vi "TAT_Auto.vi"(8 "error in (no error)":errorcluster) -> (0 "error out":errorcluster)   [LabVIEW 2017]
uses:
  Controls/TRIP_VALUS_STATUS.ctl
  <vilib>/Utility/error.llb/DialogType.ctl
  Controls/AUTO_DATA.ctl
  Controls/QUEUE_STATES.ctl
  <vilib>/Utility/miscctls.llb/LVRowAndColumnUnsignedTypeDef.ctl
  Controls/AUTO_St.ctl
  6e3b2da7-da9a-4fdb-b6c6-0a8c66529e34.vi
  da0a1603-3ba1-4d29-b87e-07a202ff7828.vi
  <vilib>/Instr/_visa.llb/VISA Configure Serial Port (Instr).vi
  Global/PLC_to_Auto.vi
  <userlib>/_OpenG.lib/array/array.llb/Search 1D Array (Boolean)__ogtk.vi
  <vilib>/Utility/config.llb/NI_LVConfig.lvlib
panel:
  out "TRIP CAUSE":T1=enum."TRIP FORCE HIGHER FAIL"
  out "TRIP FORCE":u32
  out "RESET FORCE":u32
  out "SYSTEM READY ST 2":bool
  out "CYCLE RUNNING ST 2":bool
  out "LOAD gms":cluster{"X DISTANCE":dbl[], "Y LOAD":dbl[]}(graph) caption="XY Graph - Dark"
  out "TF PART OK SCAN ST2":bool
  out "TF RUNNING PART ST2":string caption="TF RUNNING PART"
  out "LOAD":string
  out "3. POSITION 3 DONE":bool
  out "2. POSITION 2 DONE":bool
  out "1. POSITION 1 DONE":bool
  out "PART PRESENT":bool
  out "STOCK COUNTER":string
  out "MOP OPERATION OK":bool
  out "MOTOR HOME":bool
  out "PART OK ST 1":bool
  out "SYSTEM READY ST 1":bool
  out "CYCLE RUNNING STATION 1":bool
  out "Table":string[][](table)
  out "Scaned 2 Code":string
  out "Scanner 2 Status":bool
  out "mechanisum ok ack":bool
  out "housing ok ack":bool
  out "error out 2":errorcluster
  in  "COUNTER RESET":bool
  out "Load Cell Scaned":string
  out "Load Cell Status":bool
  out "Scanner 1 Status":bool
  out "Scaned 1 Code":string
  out "PLC STATUS":bool
  out "MECHANISUM DATA ST1":string caption="MECHANISUM DATA"
  out "NG COUNTER":string
  out "OK COUNTER":string
  out "CYCLE TIME (Sec)":string
  out "MAIN LOOP STOPED ?":bool
  out "Alarms":string[](array[string])
  out "HOUSING DATA ST1":string caption="HOUSING DATA"
  in  "Stop":bool
  out "DATE/TIME":string
  out "screen name":string
  out "ALARMS:-":string
  out "USER:-":string
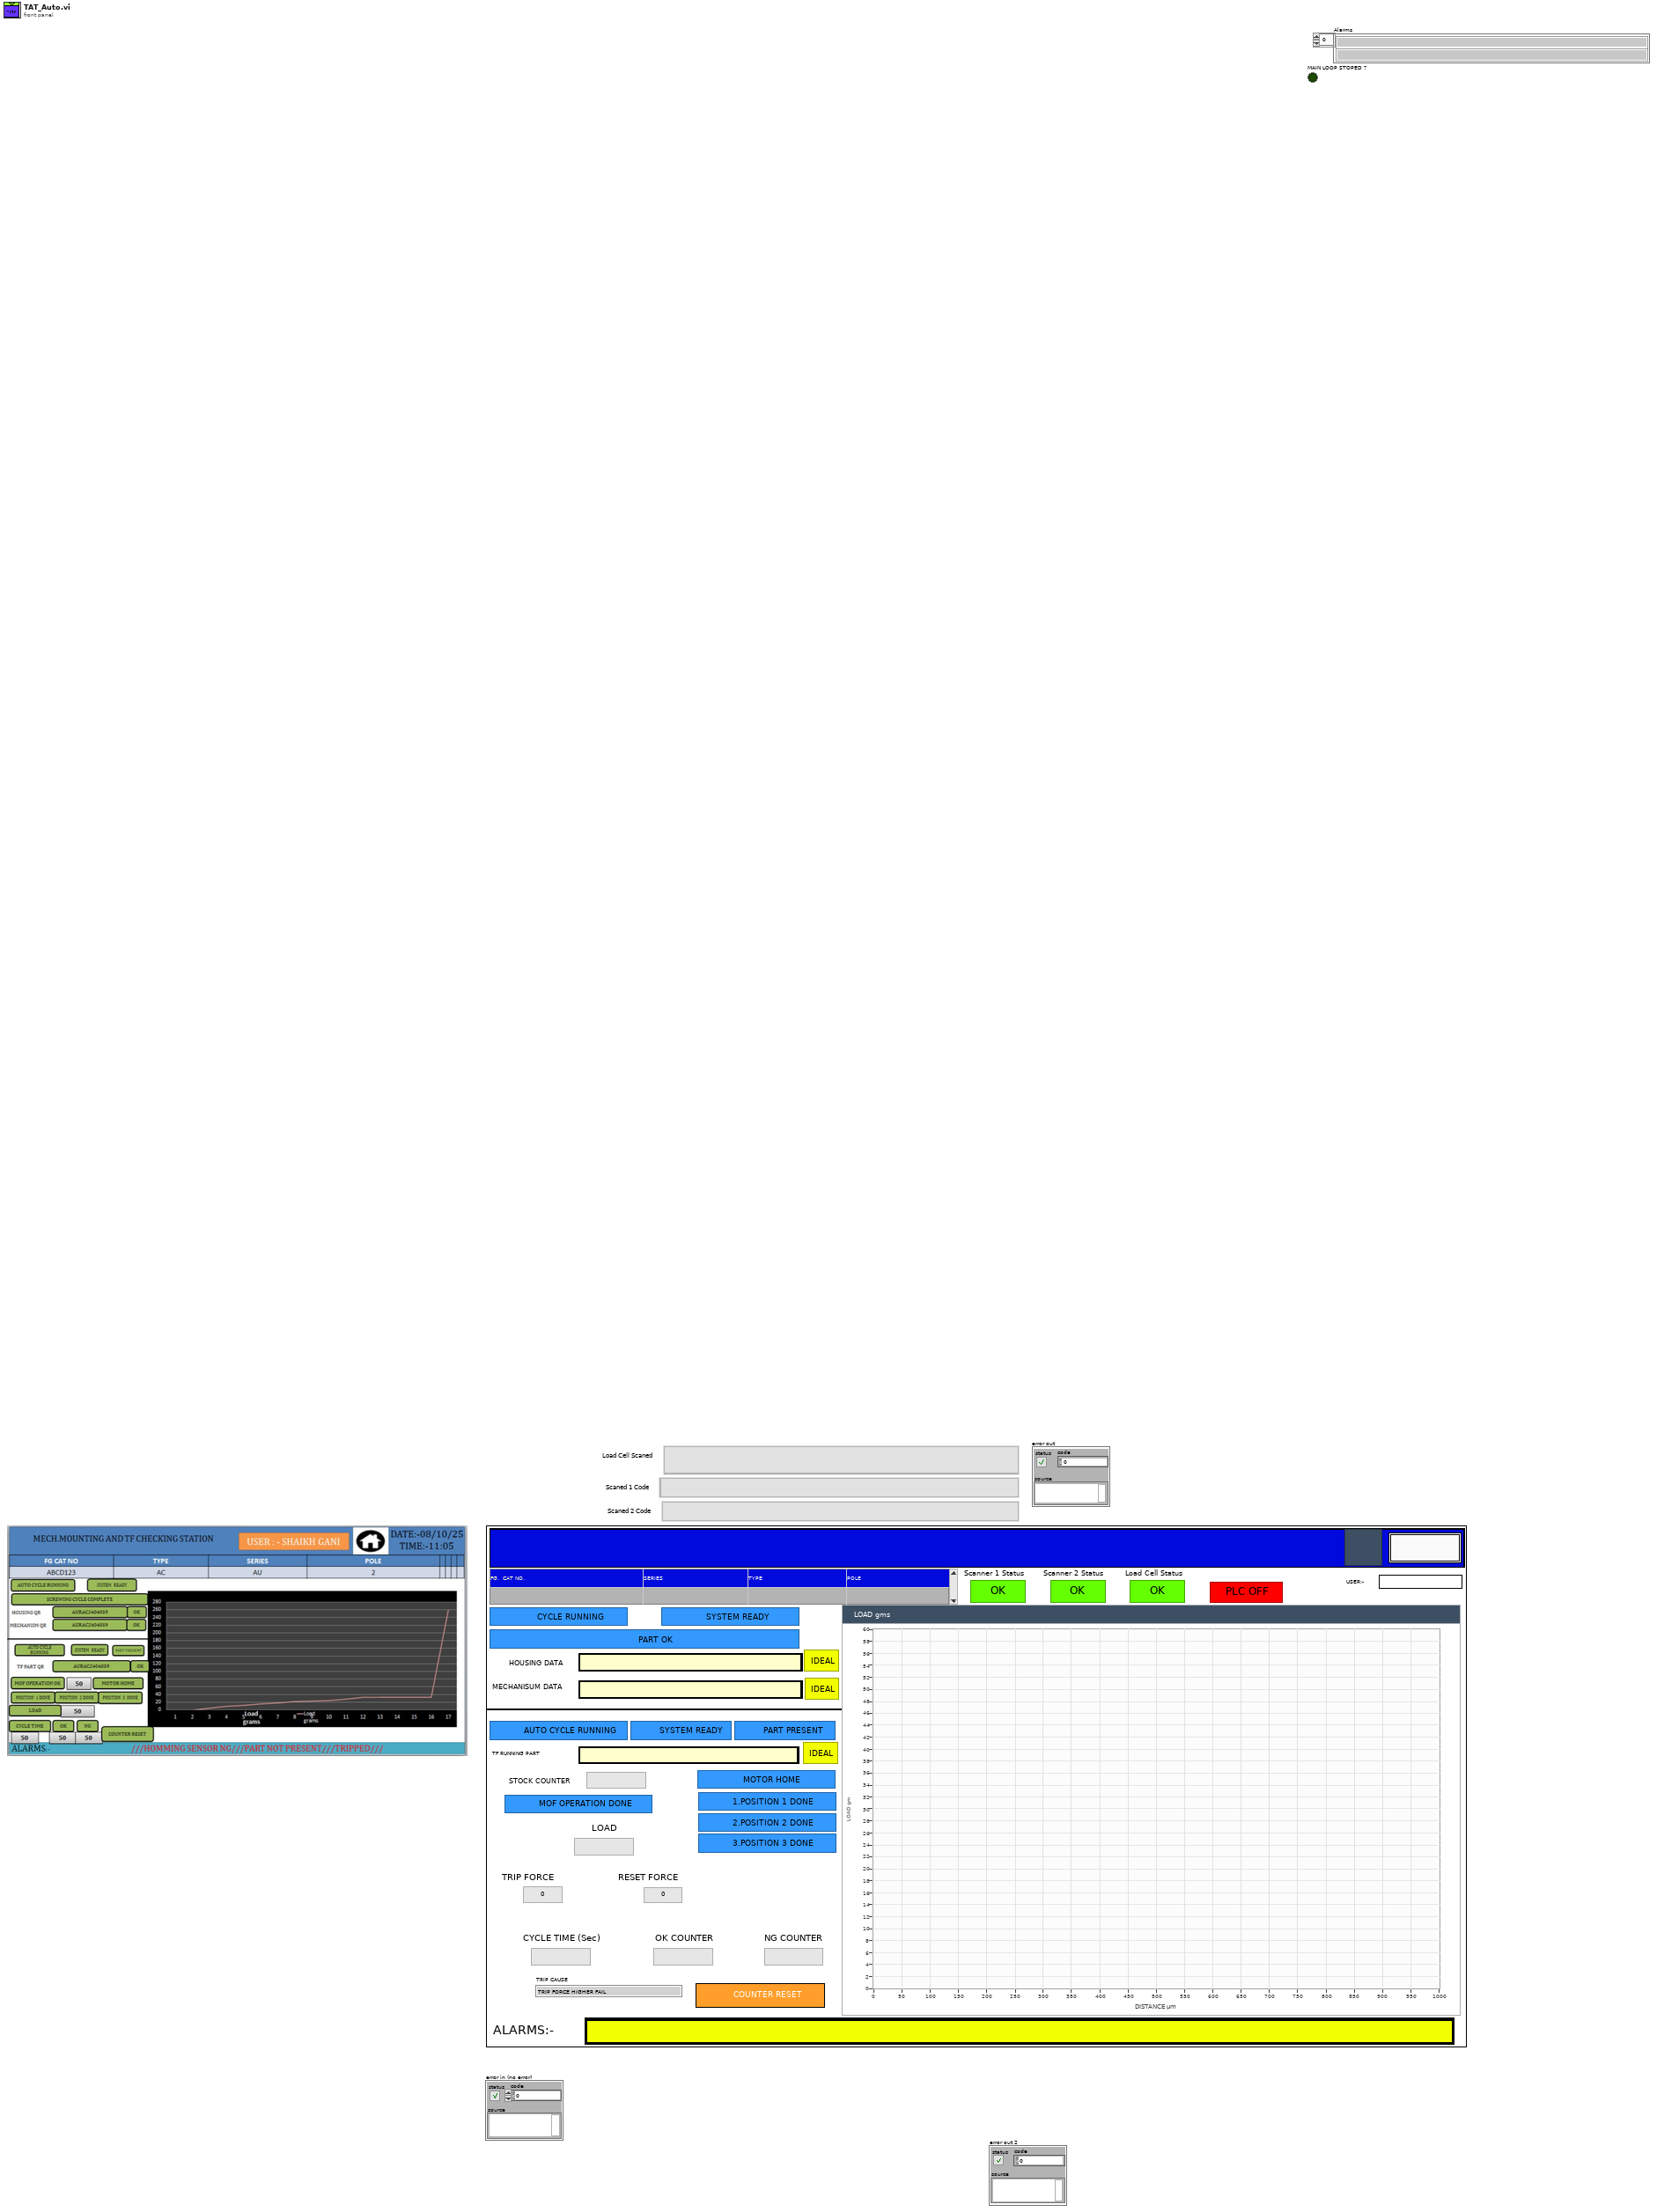
[diagram p1: front panel]
types:
  T1 = typedef "TRIP_VALUS_STATUS.ctl" = enum16{"RESET FORCE HIGHER FAIL", "TRIP FORCE HIGHER FAIL", "TRIP FORCE LOWER FAIL", "IDEAL", "TRIP RESET ACHIVED"}
  T2 = typedef "AUTO_DATA.ctl" = cluster{"SINGLE VARIENT":cluster{"HOUASING":string, "MECHANISUM":string, "VARIENT No.":string, "TYPE":string, "SERIES":string, "POLE":string}, "CYCLE DATA":cluster{"SCANNED HOUSING ST1":string, "SCANNED MECHANISUM ST1":string, "X DISTANCE":dbl[], "Y LOAD":dbl[], "prn DATA":string, "SCANNED HOUSING 1 OK":string[], "SCANNED HOUSING TF ST2":string}, "TF CHECKING PARAMATERS":cluster{"TRIP FORCE MIN":u16, "RESET FORCE MIN":u16, "OFFSET":i16, "TRIP FORCE MAX":u16, "RESET FORCE MAX":u16}, "REFERENCE":cluster{"TRIP FORCE":refnum<vi>, "RESET FORCE":refnum<vi>}}
  T3 = typedef "DialogType.ctl" = u16
  T4 = cluster{"PLC IP ADDRESS":string, "SCAN 1 COM":refnum<visa-resource-name>, "SCAN 2 COM":refnum<visa-resource-name>, "LOAD CELL COM":refnum<visa-resource-name>, "PRINTER IP ADDRESS":string}
  T5 = typedef "QUEUE_STATES.ctl" = enum16{"CREATE Q", "EN Q", "DE Q", "CLOSE Q"}
  T6 = typedef "AUTO_St.ctl" = enum16{"Int", "Int2", "CLUSTER_UPDATE", "WAIT", "AUTO_CYCLE_RUNNING_ST1", "SCAN_STATION_1", "STATION_1_CMPLT_OK", "STATION_1_ABORT_NG", "SCAN_STATION_2", "LOAD CELL PICK UP", "AUTO_CYCLE_COMP_ST2", "AUTO_CYCLE_ABORT_ST2", "PRINT", "CYCLE_DISTANCE FAIL_ST2", "AUTO_CYC_START_ST2", "Error_Handler", "Stop"}
  T7 = typedef "LVRowAndColumnUnsignedTypeDef.ctl" = cluster{"Row":u32, "Column":u32}
  T8 = enum32{"invalid app kind", "Development System", "Run Time System", "Student Edition", "Embedded LabVIEW", "Evaluation", "Custom"}
  T9 = typedef "NI_LVConfig.lvlib/Config Data RefNum.ctl" = refnum<k1>
  T10 = cluster{"HOUASING":string, "MECHANISUM":string, "VARIENT No.":string, "TYPE":string, "SERIES":string, "POLE":string}
  T11 = cluster{"TRIP FORCE MIN":u16, "RESET FORCE MIN":u16, "OFFSET":i16, "TRIP FORCE MAX":u16, "RESET FORCE MAX":u16}
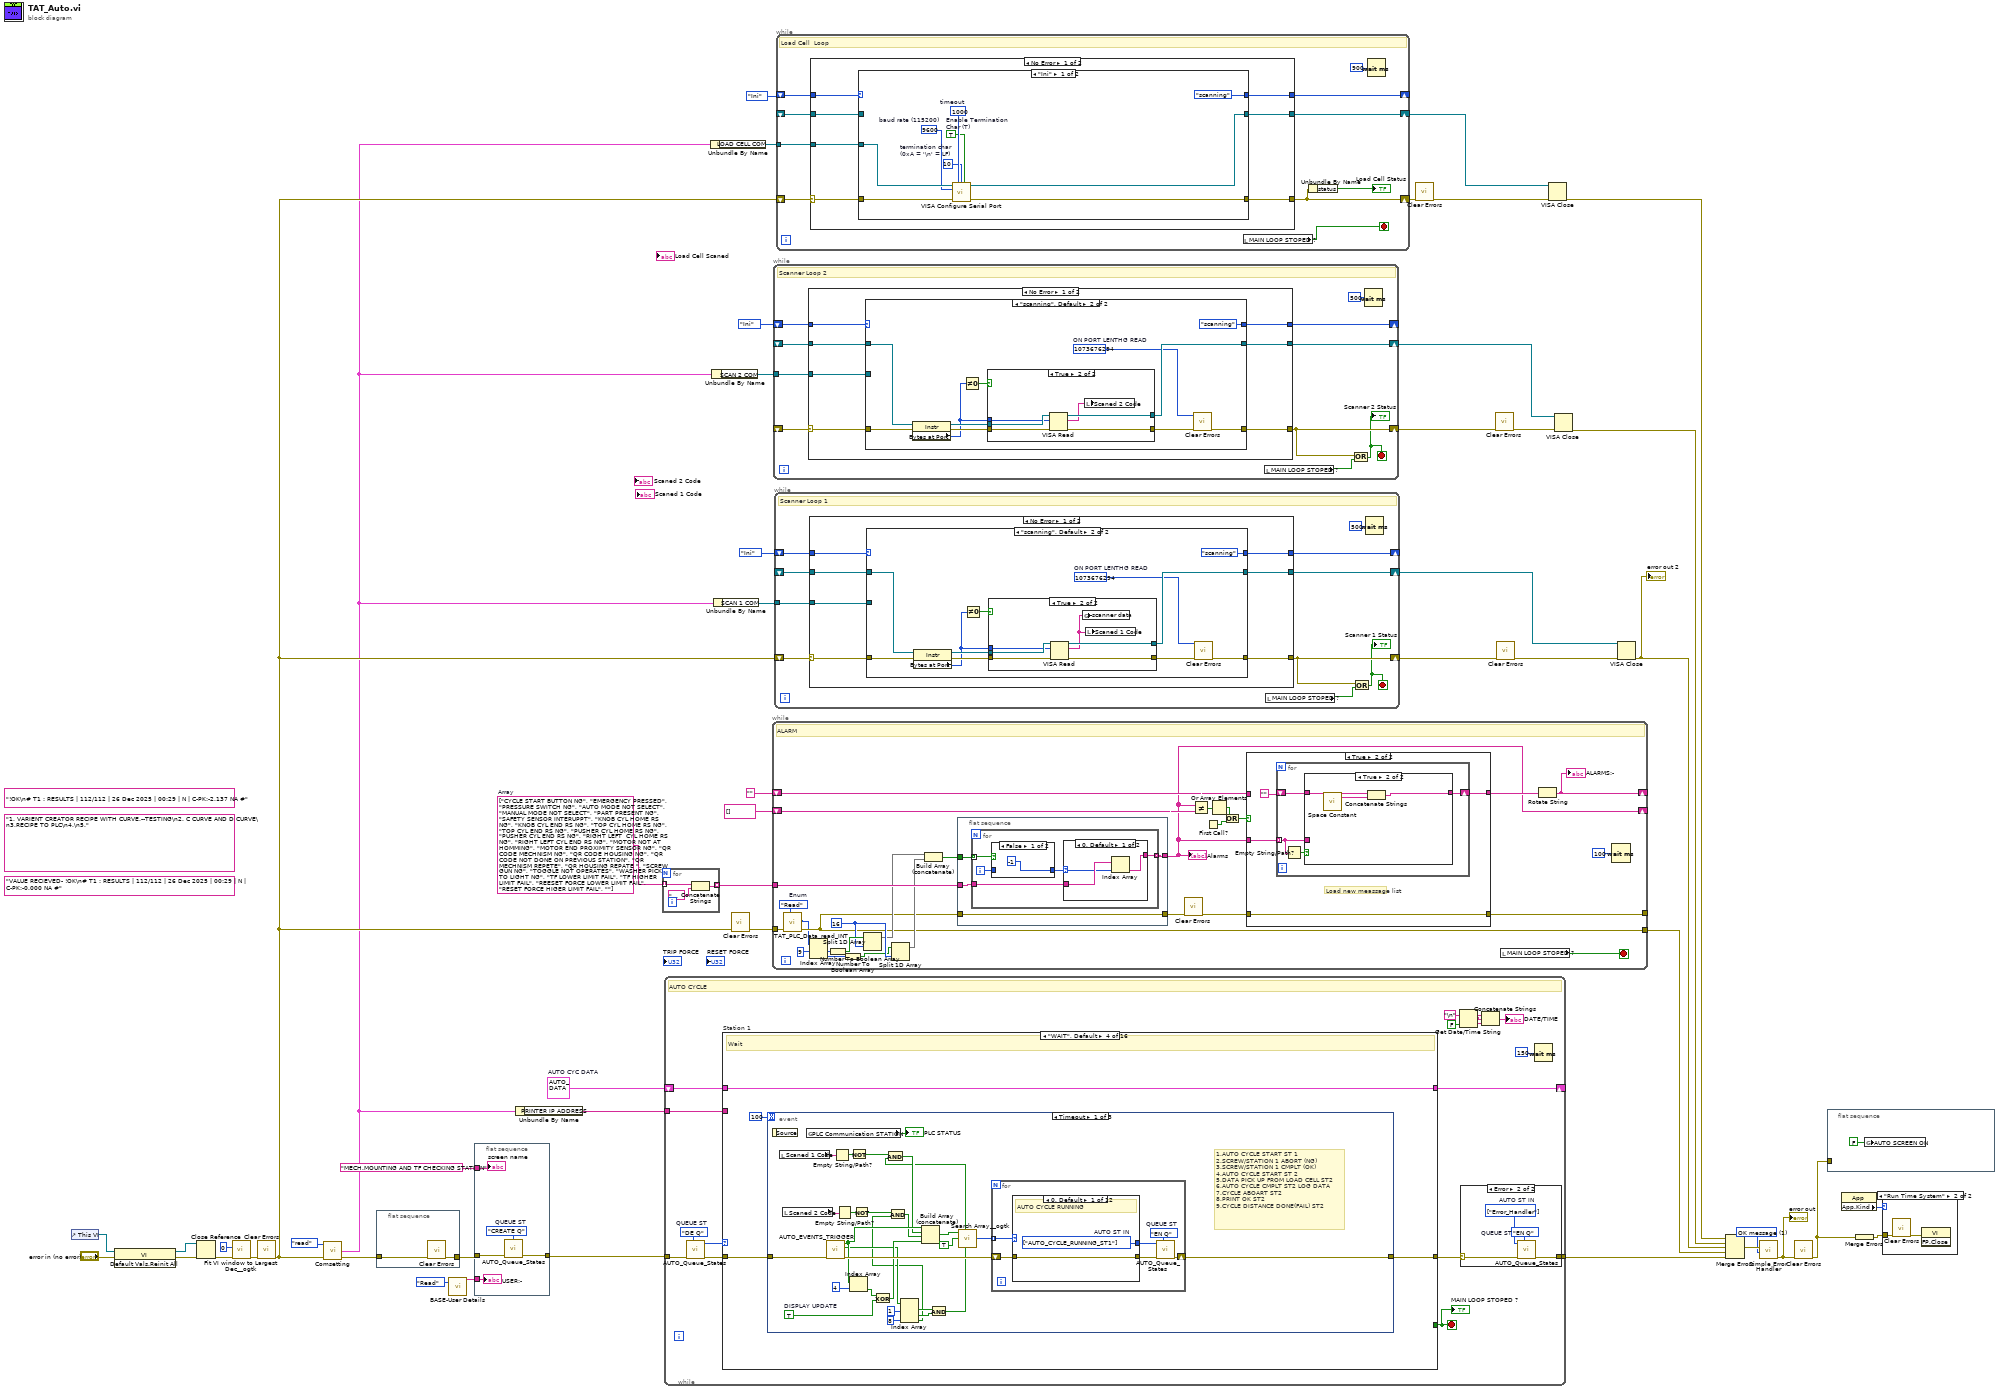
[diagram p0: block diagram]
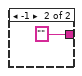
[diagram p2: hidden frame]
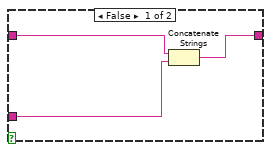
[diagram p5: hidden frame]
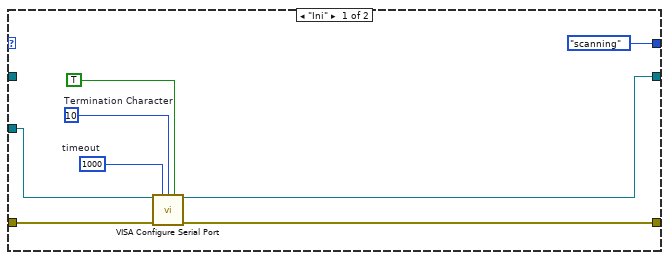
[diagram p7: hidden frame]
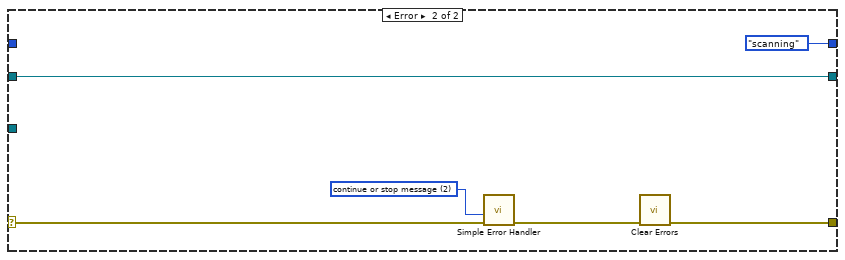
[diagram p9: hidden frame]
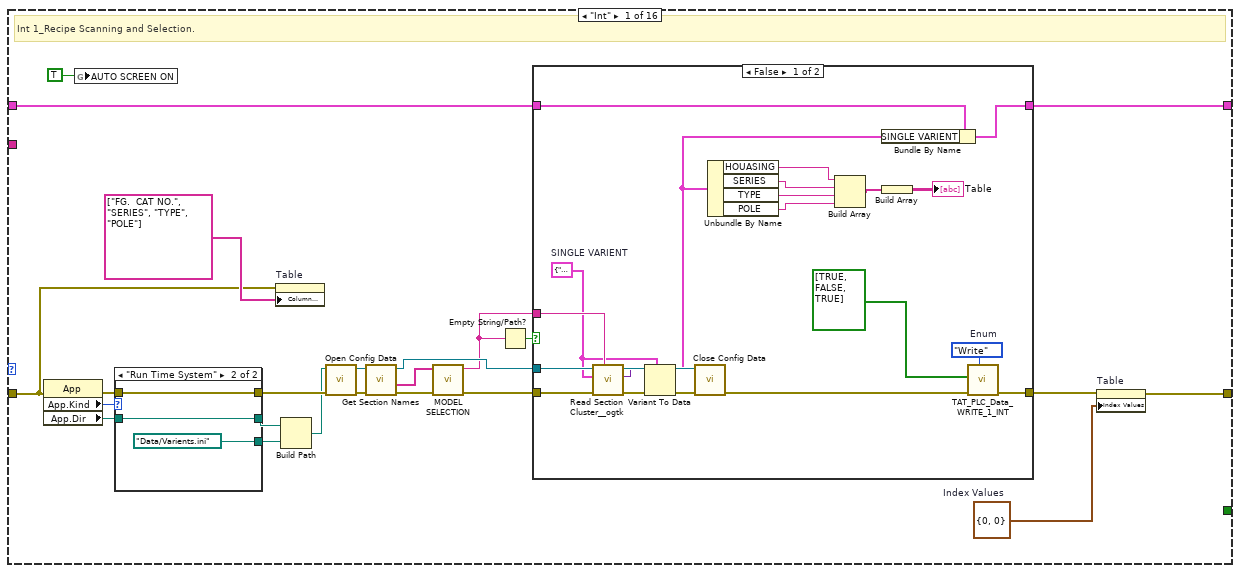
[diagram p11: hidden frame]
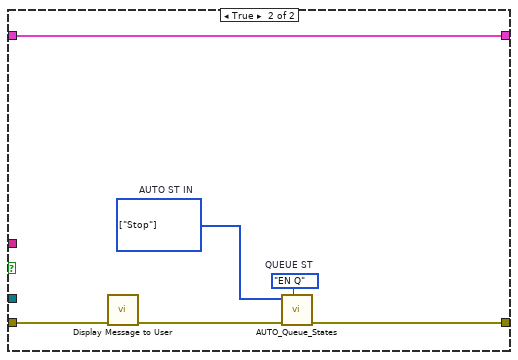
[diagram p12: hidden frame]
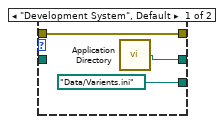
[diagram p13: hidden frame]
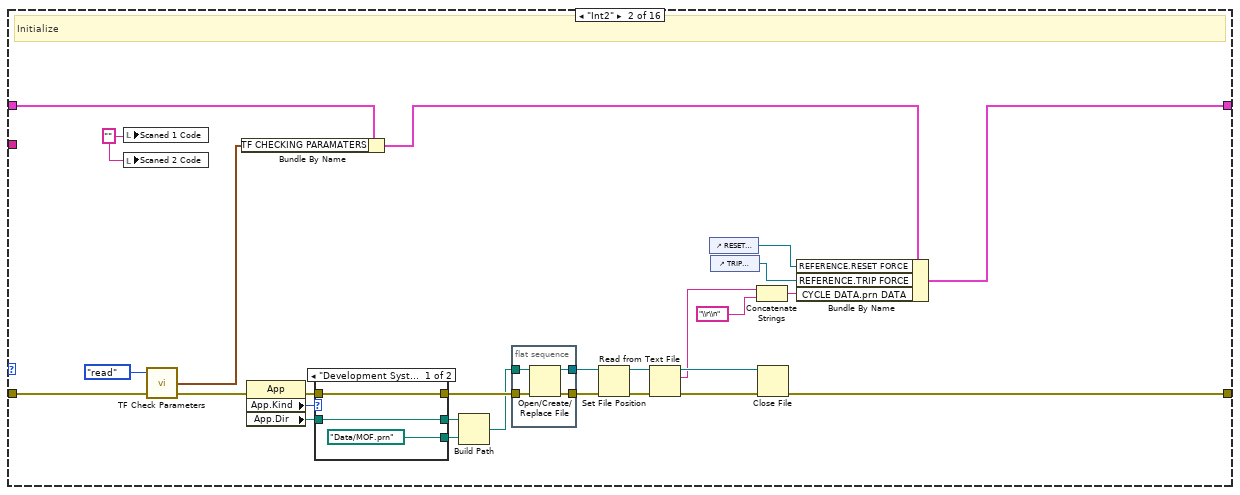
[diagram p14: hidden frame]
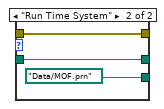
[diagram p15: hidden frame]
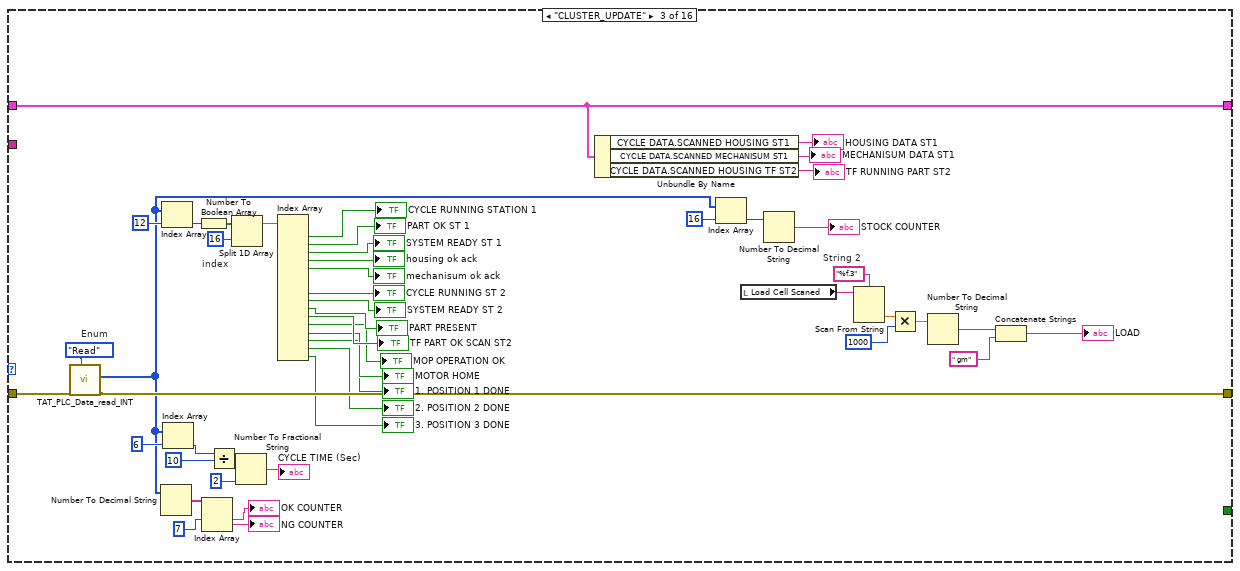
[diagram p16: hidden frame]
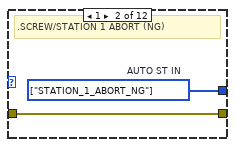
[diagram p17: hidden frame]
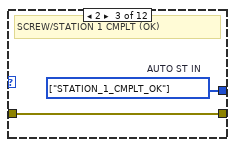
[diagram p18: hidden frame]
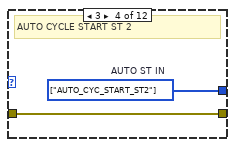
[diagram p19: hidden frame]
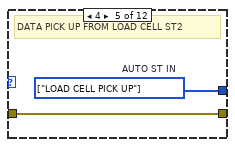
[diagram p20: hidden frame]
diagram:
  w3 = string[] ["CYCLE START BUTTON NG", "EMERGENCY PRESSED", "PRESSURE SWITCH NG", "AUTO MODE NOT SELECT", "MANUAL MODE NOT SELECT", "PART PRESENT NG", "SAFETY SENSOR INTERUPPT", "KNOB CYL HOME RS NG", "KNOB CYL END RS NG", "TOP CYL HOME RS NG", "TOP CYL END RS NG", "PUSHER CYL HOME RS NG", "PUSHER CYL END RS NG", "RIGHT LEFT  CYL HOME RS NG", "RIGHT LEFT CYL END RS NG", "MOTOR NOT AT HOMMING", "MOTOR END PROXIMITY SENSOR NG", "QR CODE MECHNISM NG", "QR CODE HOUSING NG", "QR CODE NOT DONE ON PREVIOUS STATION", "QR MECHNISM REPETE", "QR HOUSING REPATE ", "SCREW GUN NG", "TOGGLE NOT OPERATES", "WASHER PICK TO LIGHT NG", "TF LOWER LIMIT FAIL", "TF HIGHER LIMIT FAIL", "REESET FORCE LOWER LIMIT FAIL", "RESET FORCE HIGER LIMIT FAIL", ""]  # Array
  w23 = T2 {"SINGLE VARIENT"={"HOUASING"="", "MECHANISUM"="", "VARIENT No."="", "TYPE"="17.5", "SERIES"="2", "POLE"="2"}, "CYCLE DATA"={"SCANNED HOUSING ST1"="", "SCANNED MECHANISUM ST1"="", "X DISTANCE"=[], "Y LOAD"=[], "prn DATA"="", "SCANNED HOUSING 1 OK"=[], "SCANNED HOUSING TF ST2"=""}, "TF CHECKING PARAMATERS"={"TRIP FORCE MIN"=40, "RESET FORCE MIN"=350, "OFFSET"=10, "TRIP FORCE MAX"=40, "RESET FORCE MAX"=350}, "REFERENCE"={"TRIP FORCE"=refnum, "RESET FORCE"=refnum}}  # AUTO CYC DATA
  (unwired) "!OK\n# T1 : RESULTS | 112/112 | 26 Dec 2025 | 00:29 | N | C-PK:-2.137 NA #"
  (unwired) "1. VARIENT CREATOR RECIPE WITH CURVE.--TESTING\n2. C CURVE AND D CURVE\n3.RECIPE TO PLC\n4.\n5."
  (unwired) "VALUE RECIEVED- !OK\n# T1 : RESULTS | 112/112 | 26 Dec 2025 | 00:29 | N | C-PK:-0.000 NA #"
  w44 = T3 1 items=["no dialog", "OK message", "continue or stop message", "OK message + warnings", "continue/stop + warnings"] ("type of dialog (OK msg:1)")
  n1 = control-ref of="This VI"() -> (w14:refnum<vi>)
  n2 = invoke class="VI" method="Default Vals.Reinit All"(reference=w14, error in="error in (no error)") -> (reference out=w12:refnum<vi>, error out=w13:errorcluster)  [unwired: 1 in, 1 out]
  n3 = Close Reference(reference=w12, error in (no error)=w13) -> (error out=w49:errorcluster)
  n4 = call <userlib>:"Fit VI window to Largest Dec__ogtk.vi"("error in (no error)"=w49, "border spacing (2 px)"=0) -> ("error out"=w37:errorcluster)  [unwired: 4 in, 1 out]
  n5 = call <vilib>:"Clear Errors.vi"("error in (no error)"=w37) -> ("error out"=w22:errorcluster)  [unwired: 5 in, 1 out]
  n6 = call "Comsetting.vi"("error in"=w22, "Enum"=enum16{"read", "write"}."read") -> ("error our"=w26:errorcluster, "HardwareSetting"=w2:T4)  [unwired: 1 in, 1 out]
  n7 = flat-sequence {
    tunnel: [w51] -> w28
    tunnel: w26 -> [w50]
    frame #0 {
      n8 = call <vilib>:"Clear Errors.vi"("error in (no error)"=w50) -> ("error out"=w51:errorcluster)  [unwired: 5 in, 1 out]
    }
  }
  n9 = call "BASE-User Details.vi"("Enum"=enum16{"Read", "Write"}."Read") -> ("User Name Out"=w45:string)  [unwired: 9 in, 1 out]
  n10 = flat-sequence {
    tunnel: [w54] -> w39
    tunnel: w28 -> [w53]
    tunnel: w45 -> [w56]
    tunnel: "MECH.MOUNTING AND TF CHECKING STATION" -> [w52]
    frame #0 {
      w55 = QUEUE_STATES."CREATE Q"  # QUEUE ST
      n11 = call "AUTO_Queue_States.vi"("QUEUE ST"=w55, "error in"=w53) -> ("error OUT"=w54:errorcluster)  [unwired: 8 in, 1 out]
      "USER:-" <- w56
      "screen name" <- w52
    }
  }
  n12 = Unbundle By Name(w2) -> ("PRINTER IP ADDRESS"=w1:string)
  n13 = for {
    tunnel: w3 -> [w59] mode=indexing
    tunnel: [w57] -> w31 mode=indexing
    n14 = Concatenate Strings(w59, "          ") -> (w57:string)
  }
  n15 = while {
    tunnel: w39 -> [w67]
    tunnel: [w63] -> w48
    shift-right: [w61] -> _
    shift-left: w23 -> [w62]
    tunnel: w1 -> [w60]
    stop <- w69 stop-if-true
    w68 = QUEUE_STATES."DE Q"  # QUEUE ST
    # "AUTO CYCLE"
    n16 = call "AUTO_Queue_States.vi"("QUEUE ST"=w68, "error in"=w67) -> ("error OUT"=w66:errorcluster, "AUTO ST"=w65:T6)  [unwired: 8 in]
    n17 = case "Station 1" shown="\"WAIT\", Default" w65 {
      tunnel: [_ _ _ _ _ _ _ _ _ _ _ _ _ _ _ TRUE] -> w69
      tunnel: [w83 w143 w211 w225 w295 w311 w358 w362 w374 w398 w425 w445 w471 w482 w485 w494] -> w64
      tunnel: w66 -> [w81 w163 w210 w222 w295 w317 w358 w362 w375 w395 w424 w429 w471 w482 w486 w497]
      tunnel: [w86 w140 w174 w223 w293 w314 w352 w360 w372 w377 w422 w442 w464 w481 w483 w495] -> w61
      tunnel: w62 -> [w90 w161 w174 w223 w294 w319 w357 w361 w363 w376 w421 w442 w463 w480 w483 w495]
      tunnel: w60 -> [_ _ _ _ _ _ _ _ _ _ _ w444 _ _ _ _]
      frame "Int" {
        w85 = T7 {"Row"=0, "Column"=0}  # Index Values
        # "Int 1_Recipe Scanning and Selection."
        n18 = property class="App"(error in=w81) -> (error out=w99:errorcluster, "App.Kind"=w102:T8, "App.Dir"=w100:path)  [unwired: 1 in, 1 out]
        n19 = global write "PLC_to_Auto.vi" "AUTO SCREEN ON"(TRUE) -> ()
        n20 = case shown="\"Run Time System\"" w102 {
          tunnel: [w133 w136] -> w103
          tunnel: w99 -> [w133 w136]
          tunnel: w100 -> [_ w134]
          tunnel: [path "Data/Varients.ini" path "Data/Varients.ini"] -> w101
          tunnel: [w131 w134] -> w88
          frame "Development System", Default {
            n21 = call <vilib>:"Application Directory.vi"() -> ("Application Directory"=w131:path)
          }
          frame "Run Time System" {
          }
        }
        n22 = property on="Table" class="Tbl (strict)"(error in=w81, "Column Headers[]"=string[] ["FG.  CAT NO.", "SERIES", "TYPE", "POLE"]) -> ()  [unwired: 1 in, 2 out]
        n23 = Build Path(base path=w88, name or relative path=w101) -> (appended path=w89:path)
        n24 = call <vilib>:"Open Config Data.vi"("error in (no error)"=w103, "configuration file path"=w89) -> ("error out"=w98:errorcluster, "refnum"=w97:T9)  [unwired: 7 in, 1 out]
        n25 = call <vilib>:"Get Section Names.vi"("error in (no error)"=w98, "refnum"=w97) -> ("error out"=w96:errorcluster, "section names"=w95:string[], "refnum out"=w93:T9)  [unwired: 7 in]
        n26 = call "MODEL SELECTION.vi"("error in (no error)"=w96, "Plan List"=w95) -> ("error out 2"=w94:errorcluster, "SCAN ADDON CODE RECIPE"=w91:string)  [unwired: 8 in]
        n27 = Empty String/Path?(string/path=w91) -> (empty?=w92:bool)
        n28 = case shown="False" w92 {
          tunnel: w94 -> [w124 w129]
          tunnel: [w113 w126] -> w84
          tunnel: w93 -> [w122 _]
          tunnel: w91 -> [w121 _]
          tunnel: [w116 w130] -> w86
          tunnel: w90 -> [w117 w130]
          frame False {
            w110 = T10 {"HOUASING"="", "MECHANISUM"="", "VARIENT No."="", "TYPE"="", "SERIES"="", "POLE"="2"}  # SINGLE VARIENT
            w115 = enum16{"Read", "Write"}."Write"  # Enum
            n29 = call <userlib>:"Read Section Cluster__ogtk.vi"("section (optional)"=w121, "error in (no error)"=w124, "Section Formatted Cluster Type"=w110, "refnum"=w122) -> ("error out"=w120:errorcluster, "Section Formatted Cluster"=w118:variant, "dup refnum"=w123:T9)  [unwired: 3 in, 2 out]
            n30 = Variant To Data(error in=w120, type=w110, Variant=w118) -> (data=w111:T10, error out=w119:errorcluster)
            n31 = call <vilib>:"Close Config Data.vi"("error in (no error)"=w119, "refnum"=w123) -> ("error out"=w114:errorcluster)  [unwired: 8 in, 1 out]
            n32 = Unbundle By Name(w111) -> ("HOUASING"=w109:string, "SERIES"=w107:string, "TYPE"=w106:string, "POLE"=w105:string)
            n33 = Build Array(w109, w107, w106, w105) -> (w108:string[])
            n34 = Bundle By Name(cluster=w117, "SINGLE VARIENT"=w111) -> (w116:T2)
            n35 = Build Array(w108) -> (→"Table":string[][])
            n36 = call "TAT_PLC_Data_WRITE_1_INT.vi"("Enum"=w115, "error in (no error)"=w114, "Array"=bool[] [TRUE, FALSE, TRUE]) -> ("error out"=w113:errorcluster)  [unwired: 7 in, 1 out]
          }
          frame True {
            w125 = T6[] [enum."Stop"] items=["Int", "Int2", "CLUSTER_UPDATE", "WAIT", "AUTO_CYCLE_RUNNING_ST1", "SCAN_STATION_1", "STATION_1_CMPLT_OK", "STATION_1_ABORT_NG", "SCAN_STATION_2", "LOAD CELL PICK UP", "AUTO_CYCLE_COMP_ST2", "AUTO_CYCLE_ABORT_ST2", "PRINT", "CYCLE_DISTANCE FAIL_ST2", "AUTO_CYC_START_ST2", "Error_Handler", "Stop"]  # AUTO ST IN
            w128 = QUEUE_STATES."EN Q"  # QUEUE ST
            n37 = call "Display Message to User"("error in (no error)"=w129) -> ("error out"=w127:errorcluster)  [unwired: 9 in, 1 out]
            n38 = call "AUTO_Queue_States.vi"("QUEUE ST"=w128, "error in"=w127, "AUTO ST IN"=w125) -> ("error OUT"=w126:errorcluster)  [unwired: 7 in, 1 out]
          }
        }
        n39 = property on="Table" class="Tbl (strict)"(error in=w84, "Index Values"=w85) -> (error out=w83:errorcluster)  [unwired: 1 in, 1 out]
      }
      frame "Int2" {
        w139 = ""
        # "Initialize"
        n40 = local write "Scaned 1 Code"(w139) -> ()
        n41 = local write "Scaned 2 Code"(w139) -> ()
        n42 = call "TF Check Parameters.vi"("error in"=w163, "Enum"=enum16{"read", "write"}."read") -> ("error our"=w144:errorcluster, "TF CHECKING PARAMATERS OUT"=w160:T11)  [unwired: 1 in, 1 out]
        n43 = Bundle By Name(cluster=w161, "TF CHECKING PARAMATERS"=w160) -> (w141:T2)
        n44 = property class="App"(error in=w144) -> (error out=w149:errorcluster, "App.Kind"=w147:T8, "App.Dir"=w148:path)  [unwired: 1 in, 1 out]
        n45 = case shown="\"Development System\", Default" w147 {
          tunnel: [w166 w169] -> w146
          tunnel: w149 -> [w166 w169]
          tunnel: w148 -> [w164 w168]
          tunnel: [w164 w168] -> w150
          tunnel: [path "Data/MOF.prn" path "Data/MOF.prn"] -> w151
          frame "Development System", Default {
          }
          frame "Run Time System" {
          }
        }
        n46 = Build Path(base path=w150, name or relative path=w151) -> (appended path=w145:path)
        n47 = flat-sequence {
          tunnel: w146 -> [w173]
          tunnel: [w172] -> w155
          tunnel: [w171] -> w153
          tunnel: w145 -> [w170]
          frame #0 {
            n48 = Open/Create/Replace File(file path (use dialog)=w170, error in=w173) -> (refnum out=w171:refnum<file>, error out=w172:errorcluster)  [unwired: 4 in, 1 out]
          }
        }
        n49 = Set File Position(refnum=w153, error in=w155) -> (refnum out=w152:refnum<file>, error out=w154:errorcluster)  [unwired: 2 in]
        n50 = Read from Text File(file (use dialog)=w152, error in=w154) -> (refnum out=w159:refnum<file>, text=w156:string, error out=w158:errorcluster)  [unwired: 2 in, 1 out]
        n51 = control-ref of="RESET FORCE"() -> (w137:refnum<vi>)
        n52 = control-ref of="TRIP FORCE"() -> (w138:refnum<vi>)
        n53 = Concatenate Strings(w156, "\\r\\n") -> (w142:string)
        n54 = Close File(refnum=w159, error in=w158) -> (error out=w143:errorcluster)  [unwired: 1 out]
        n55 = Bundle By Name(cluster=w141, "REFERENCE.RESET FORCE"=w137, "REFERENCE.TRIP FORCE"=w138, "CYCLE DATA.prn DATA"=w142) -> (w140:T2)
      }
      frame "CLUSTER_UPDATE" {
        w196 = "%f.3"  # String 2
        w208 = 16  # index
        w212 = enum16{"Read", "Write"}."Read"  # Enum
        n56 = call "TAT_PLC_Data_read_INT.vi"("Enum"=w212, "error in (no error)"=w210) -> ("error out"=w211:errorcluster, "Array 2"=w192:u16[])  [unwired: 8 in]
        n57 = Number To Decimal String(number=w192) -> (decimal integer string=w221:string[])  [unwired: 1 in]
        n58 = Index Array(array=w192, index=12) -> (element=w206:u16)
        n59 = Index Array(array=w192, index=6) -> (element=w218:u16)
        n60 = Number To Boolean Array(number=w206) -> (Boolean array=w207:bool[])
        n61 = Index Array(array=w221, index #1=7) -> (element #1=→"OK COUNTER":string, element #2=→"NG COUNTER":string)  [unwired: 1 in]
        n62 = Divide(x=w218, y=10) -> (x/y=w217:dbl)
        n63 = Split 1D Array(array=w207, index=w208) -> (first subarray=w209:bool[])  [unwired: 1 out]
        n64 = Number To Fractional String(number=w217, precision (6)=2) -> (F-format string=→"CYCLE TIME (Sec)":string)  [unwired: 2 in]
        n65 = Index Array(array=w209) -> (element #1=→"CYCLE RUNNING STATION 1":bool, element #2=→"PART OK ST 1":bool, element #3=→"SYSTEM READY ST 1":bool, element #4=→"housing ok ack":bool, element #5=→"mechanisum ok ack":bool, element #8=→"CYCLE RUNNING ST 2":bool, element #9=→"SYSTEM READY ST 2":bool, element #10=→"PART PRESENT":bool, element #11=→"TF PART OK SCAN ST2":bool, element #12=→"MOP OPERATION OK":bool, element #13=→"MOTOR HOME":bool, element #14=→"1. POSITION 1 DONE":bool, element #15=→"2. POSITION 2 DONE":bool, element #16=→"3. POSITION 3 DONE":bool)  [unwired: 16 in, 2 out]
        n66 = Unbundle By Name(w174) -> ("CYCLE DATA.SCANNED HOUSING ST1"=→"HOUSING DATA ST1":string, "CYCLE DATA.SCANNED MECHANISUM ST1"=→"MECHANISUM DATA ST1":string, "CYCLE DATA.SCANNED HOUSING TF ST2"=→"TF RUNNING PART ST2":string)
        n67 = Index Array(array=w192, index=16) -> (element=w191:u16)
        n68 = local read "Load Cell Scaned"() -> (w194:string)
        n69 = Number To Decimal String(number=w191) -> (decimal integer string=→"STOCK COUNTER":string)  [unwired: 1 in]
        n70 = Scan From String(format string=w196, input string=w194) -> (output 1=w197:dbl)  [unwired: 3 in, 3 out]
        n71 = Multiply(x=w197, y=1000) -> (x*y=w195:dbl)
        n72 = Number To Decimal String(number=w195) -> (decimal integer string=w188:string)  [unwired: 1 in]
        n73 = Concatenate Strings(w188, " gm") -> (→"LOAD":string)
      }
      frame "WAIT", Default {
        # "Wait"
        n74 = event shown="[0] Timeout" {
          selector: _ -> [_ _ _]
          dyn-events: _ -> [_ _ _]
          timeout: 100 -> [_ _ _]
          tunnel: [w246 w284 w288] -> w225
          tunnel: w222 -> [w252 w283 w289]
          event Timeout {
            w241 = TRUE  # DISPLAY UPDATE
            # "1.AUTO CYCLE START ST 1\n2.SCREW/STATION 1 ABORT (NG)\n3.SCREW/STATION 1 CMPLT (OK)\n4.AUTO CYCLE START ST 2\n5.DATA PICK UP FROM LOAD CELL ST2\n6.AUTO CYCLE CMPLT ST2 LOG DATA\n7.CYCLE ABOART ST2\n8.PRINT OK ST2\n9.CYCLE DISTANCE DONE(FAIL) ST2"
            n75 = event-data() -> ()  [unwired: 1 in, 1 out]
            n76 = local read "Scaned 1 Code"() -> (w233:string)
            n77 = local read "Scaned 2 Code"() -> (w245:string)
            n78 = global read "PLC_to_Auto.vi" "PLC Communication STATION 1"() -> (→"PLC STATUS":bool)
            n79 = call "AUTO_EVENTS_TRIGGER.vi"("error in"=w252) -> ("error out"=w250:errorcluster, "raw array"=w231:bool[], "Array"=w244:bool[])  [unwired: 8 in]
            n80 = Empty String/Path?(string/path=w233) -> (empty?=w235:bool)
            n81 = Empty String/Path?(string/path=w245) -> (empty?=w239:bool)
            n82 = Index Array(array=w244, index=4) -> (element=w242:bool)
            n83 = Not(x=w235) -> (.not. x?=w236:bool)
            n84 = Not(x=w239) -> (.not. x?=w238:bool)
            n85 = Exclusive Or(1:w241, 2:w242) -> (0:w240:bool)
            n86 = Index Array(array=w231, index #1=1, index #3=8) -> (element #1=w229:bool, element #2=w228:bool, element #3=w227:bool)  [unwired: 1 in]
            n87 = And(x=w238, y=w227) -> (x .and. y?=w237:bool)
            n88 = And(x=w229, y=w228) -> (x .and. y?=w232:bool)
            n89 = And(x=w236, y=w232) -> (x .and. y?=w234:bool)
            n90 = Build Array (concatenate)(w244, w234, w237, w240) -> (w248:bool[])
            n91 = call-poly <userlib>:"Search Array__ogtk.vi"("Array"=w248, "Element Data"=TRUE) -> ("Indices of Elements"=w251:i32[])  [unwired: 7 in]
            n92 = for {
              tunnel: w251 -> [w258] mode=indexing
              shift-right: [w257] -> w246
              shift-left: w250 -> [w254]
              w256 = QUEUE_STATES."EN Q"  # QUEUE ST
              n93 = case shown="0, Default" w258 {
                tunnel: [w260 w262 w264 w266 w268 w270 w272 w274 w276 w278 w280 w282] -> w255
                tunnel: w254 -> [w260 w262 w264 w266 w268 w270 w272 w274 w276 w278 w280 w282]
                tunnel: [w259 w261 w263 w265 w267 w269 w271 w273 w275 w277 w279 w281] -> w253
                frame 0, Default {
                  w259 = T6[] [enum."AUTO_CYCLE_RUNNING_ST1"] items=["Int", "Int2", "CLUSTER_UPDATE", "WAIT", "AUTO_CYCLE_RUNNING_ST1", "SCAN_STATION_1", "STATION_1_CMPLT_OK", "STATION_1_ABORT_NG", "SCAN_STATION_2", "LOAD CELL PICK UP", "AUTO_CYCLE_COMP_ST2", "AUTO_CYCLE_ABORT_ST2", "PRINT", "CYCLE_DISTANCE FAIL_ST2", "AUTO_CYC_START_ST2", "Error_Handler", "Stop"]  # AUTO ST IN
                  # "AUTO CYCLE RUNNING"
                }
                frame 1 {
                  w261 = T6[] [enum."STATION_1_ABORT_NG"] items=["Int", "Int2", "CLUSTER_UPDATE", "WAIT", "AUTO_CYCLE_RUNNING_ST1", "SCAN_STATION_1", "STATION_1_CMPLT_OK", "STATION_1_ABORT_NG", "SCAN_STATION_2", "LOAD CELL PICK UP", "AUTO_CYCLE_COMP_ST2", "AUTO_CYCLE_ABORT_ST2", "PRINT", "CYCLE_DISTANCE FAIL_ST2", "AUTO_CYC_START_ST2", "Error_Handler", "Stop"]  # AUTO ST IN
                  # ".SCREW/STATION 1 ABORT (NG)"
                }
                frame 2 {
                  w263 = T6[] [enum."STATION_1_CMPLT_OK"] items=["Int", "Int2", "CLUSTER_UPDATE", "WAIT", "AUTO_CYCLE_RUNNING_ST1", "SCAN_STATION_1", "STATION_1_CMPLT_OK", "STATION_1_ABORT_NG", "SCAN_STATION_2", "LOAD CELL PICK UP", "AUTO_CYCLE_COMP_ST2", "AUTO_CYCLE_ABORT_ST2", "PRINT", "CYCLE_DISTANCE FAIL_ST2", "AUTO_CYC_START_ST2", "Error_Handler", "Stop"]  # AUTO ST IN
                  # "SCREW/STATION 1 CMPLT (OK)"
                }
                frame 3 {
                  w265 = T6[] [enum."AUTO_CYC_START_ST2"] items=["Int", "Int2", "CLUSTER_UPDATE", "WAIT", "AUTO_CYCLE_RUNNING_ST1", "SCAN_STATION_1", "STATION_1_CMPLT_OK", "STATION_1_ABORT_NG", "SCAN_STATION_2", "LOAD CELL PICK UP", "AUTO_CYCLE_COMP_ST2", "AUTO_CYCLE_ABORT_ST2", "PRINT", "CYCLE_DISTANCE FAIL_ST2", "AUTO_CYC_START_ST2", "Error_Handler", "Stop"]  # AUTO ST IN
                  # "AUTO CYCLE START ST 2"
                }
                frame 4 {
                  w267 = T6[] [enum."LOAD CELL PICK UP"] items=["Int", "Int2", "CLUSTER_UPDATE", "WAIT", "AUTO_CYCLE_RUNNING_ST1", "SCAN_STATION_1", "STATION_1_CMPLT_OK", "STATION_1_ABORT_NG", "SCAN_STATION_2", "LOAD CELL PICK UP", "AUTO_CYCLE_COMP_ST2", "AUTO_CYCLE_ABORT_ST2", "PRINT", "CYCLE_DISTANCE FAIL_ST2", "AUTO_CYC_START_ST2", "Error_Handler", "Stop"]  # AUTO ST IN
                  # "DATA PICK UP FROM LOAD CELL ST2"
                }
                frame 5 {
                  w269 = T6[] [enum."AUTO_CYCLE_COMP_ST2"] items=["Int", "Int2", "CLUSTER_UPDATE", "WAIT", "AUTO_CYCLE_RUNNING_ST1", "SCAN_STATION_1", "STATION_1_CMPLT_OK", "STATION_1_ABORT_NG", "SCAN_STATION_2", "LOAD CELL PICK UP", "AUTO_CYCLE_COMP_ST2", "AUTO_CYCLE_ABORT_ST2", "PRINT", "CYCLE_DISTANCE FAIL_ST2", "AUTO_CYC_START_ST2", "Error_Handler", "Stop"]  # AUTO ST IN
                  # "AUTO CYCLE CMPLT ST2 LOG DATA"
                }
                frame 6 {
                  w271 = T6[] [enum."AUTO_CYCLE_ABORT_ST2"] items=["Int", "Int2", "CLUSTER_UPDATE", "WAIT", "AUTO_CYCLE_RUNNING_ST1", "SCAN_STATION_1", "STATION_1_CMPLT_OK", "STATION_1_ABORT_NG", "SCAN_STATION_2", "LOAD CELL PICK UP", "AUTO_CYCLE_COMP_ST2", "AUTO_CYCLE_ABORT_ST2", "PRINT", "CYCLE_DISTANCE FAIL_ST2", "AUTO_CYC_START_ST2", "Error_Handler", "Stop"]  # AUTO ST IN
                  # "CYCLE ABOART ST2"
                }
                frame 7 {
                  w273 = T6[] [enum."PRINT"] items=["Int", "Int2", "CLUSTER_UPDATE", "WAIT", "AUTO_CYCLE_RUNNING_ST1", "SCAN_STATION_1", "STATION_1_CMPLT_OK", "STATION_1_ABORT_NG", "SCAN_STATION_2", "LOAD CELL PICK UP", "AUTO_CYCLE_COMP_ST2", "AUTO_CYCLE_ABORT_ST2", "PRINT", "CYCLE_DISTANCE FAIL_ST2", "AUTO_CYC_START_ST2", "Error_Handler", "Stop"]  # AUTO ST IN
                  # "PRINT OK ST2"
                }
                frame 8 {
                  w275 = T6[] [enum."CYCLE_DISTANCE FAIL_ST2"] items=["Int", "Int2", "CLUSTER_UPDATE", "WAIT", "AUTO_CYCLE_RUNNING_ST1", "SCAN_STATION_1", "STATION_1_CMPLT_OK", "STATION_1_ABORT_NG", "SCAN_STATION_2", "LOAD CELL PICK UP", "AUTO_CYCLE_COMP_ST2", "AUTO_CYCLE_ABORT_ST2", "PRINT", "CYCLE_DISTANCE FAIL_ST2", "AUTO_CYC_START_ST2", "Error_Handler", "Stop"]  # AUTO ST IN
                  # "CYCLE DISTANCE DONE(FAIL) ST2"
                }
                frame 9 {
                  w277 = T6[] [enum."SCAN_STATION_1"] items=["Int", "Int2", "CLUSTER_UPDATE", "WAIT", "AUTO_CYCLE_RUNNING_ST1", "SCAN_STATION_1", "STATION_1_CMPLT_OK", "STATION_1_ABORT_NG", "SCAN_STATION_2", "LOAD CELL PICK UP", "AUTO_CYCLE_COMP_ST2", "AUTO_CYCLE_ABORT_ST2", "PRINT", "CYCLE_DISTANCE FAIL_ST2", "AUTO_CYC_START_ST2", "Error_Handler", "Stop"]  # AUTO ST IN
                  # "SCAN STATION 1"
                }
                frame 10 {
                  w279 = T6[] [enum."SCAN_STATION_2"] items=["Int", "Int2", "CLUSTER_UPDATE", "WAIT", "AUTO_CYCLE_RUNNING_ST1", "SCAN_STATION_1", "STATION_1_CMPLT_OK", "STATION_1_ABORT_NG", "SCAN_STATION_2", "LOAD CELL PICK UP", "AUTO_CYCLE_COMP_ST2", "AUTO_CYCLE_ABORT_ST2", "PRINT", "CYCLE_DISTANCE FAIL_ST2", "AUTO_CYC_START_ST2", "Error_Handler", "Stop"]  # AUTO ST IN
                  # "SCAN STATION 2"
                }
                frame 11 {
                  w281 = T6[] [enum."CLUSTER_UPDATE"] items=["Int", "Int2", "CLUSTER_UPDATE", "WAIT", "AUTO_CYCLE_RUNNING_ST1", "SCAN_STATION_1", "STATION_1_CMPLT_OK", "STATION_1_ABORT_NG", "SCAN_STATION_2", "LOAD CELL PICK UP", "AUTO_CYCLE_COMP_ST2", "AUTO_CYCLE_ABORT_ST2", "PRINT", "CYCLE_DISTANCE FAIL_ST2", "AUTO_CYC_START_ST2", "Error_Handler", "Stop"]  # AUTO ST IN
                  # "CLUSTER UPDATE"
                }
              }
              n94 = call "AUTO_Queue_States.vi"("QUEUE ST"=w256, "error in"=w255, "AUTO ST IN"=w253) -> ("error OUT"=w257:errorcluster)  [unwired: 7 in, 1 out]
            }
          }
          event "Stop": Value Change {
            w285 = QUEUE_STATES."EN Q"  # QUEUE ST
            n95 = event-data() -> ()  [unwired: 1 in, 1 out]
            n96 = Build Array(AUTO_St."Stop" ("Unload ST")) -> (w287:T6[])
            n97 = call "AUTO_Queue_States.vi"("QUEUE ST"=w285, "error in"=w283, "AUTO ST IN"=w287) -> ("error OUT"=w284:errorcluster)  [unwired: 7 in, 1 out]
          }
          event "COUNTER RESET": Value Change {
            w291 = enum16{"Read", "Write"}."Write"  # Enum
            w290 = bool[] [FALSE, FALSE, FALSE, FALSE, FALSE, FALSE, FALSE, FALSE, FALSE, FALSE, FALSE, FALSE, TRUE, FALSE, FALSE, FALSE, FALSE, FALSE, FALSE, FALSE, FALSE, FALSE, FALSE, FALSE, FALSE, FALSE, FALSE, FALSE, FALSE, FALSE, FALSE, FALSE]  # robo stop
            n98 = event-data() -> ()  [unwired: 1 in, 6 out]
            n99 = call "TAT_PLC_Data_WRITE_2_INT.vi"("Enum"=w291, "error in (no error)"=w289, "Array"=w290) -> ("error out"=w288:errorcluster)  [unwired: 7 in, 1 out]
          }
        }
      }
      frame "AUTO_CYCLE_RUNNING_ST1" {
        w292 = ""
        n100 = Bundle By Name(cluster=w294, "CYCLE DATA.SCANNED MECHANISUM ST1"=w292, "CYCLE DATA.SCANNED HOUSING ST1"=w292) -> (w293:T2)
        n101 = local write "MECHANISUM DATA ST1"(w292) -> ()
        n102 = local write "HOUSING DATA ST1"(w292) -> ()
        n103 = local write "Scaned 1 Code"(w292) -> ()
      }
      frame "SCAN_STATION_1" {
        w305 = 16  # index
        w304 = enum16{"Read", "Write"}."Read"  # Enum
        w313 = enum16{"Read", "Write"}."Write"  # Enum
        # "STATION 1 SCANNING"
        n104 = flat-sequence {
          tunnel: [w327] -> w318
          tunnel: w317 -> [w327]
          tunnel: [w326] -> w315
          tunnel: [w330] -> w302
          tunnel: w318 -> [w330]
          tunnel: [w329] -> w316
          tunnel: w315 -> [w329]
          frame #0 {
            n105 = local read "Scaned 1 Code"() -> (w326:string)
          }
          frame #1 {
            n106 = local write "Scaned 1 Code"("") -> ()
          }
        }
        n107 = Unbundle By Name(w319) -> ("SINGLE VARIENT.HOUASING"=w323:string, "SINGLE VARIENT.MECHANISUM"=w325:string)
        n108 = String Length(string=w325) -> (length=w321:i32)
        n109 = String Length(string=w323) -> (length=w320:i32)
        n110 = call "TAT_PLC_Data_read_INT.vi"("Enum"=w304, "error in (no error)"=w302) -> ("error out"=w301:errorcluster, "Array 2"=w309:u16[])  [unwired: 8 in]
        n111 = String Subset(string=w316, length (rest)=w321) -> (substring=w324:string)  [unwired: 1 in]
        n112 = String Subset(string=w316, length (rest)=w320) -> (substring=w322:string)  [unwired: 1 in]
        n113 = Index Array(array=w309) -> (element=w308:u16)  [unwired: 1 in]
        n114 = Equal?(x=w322, y=w323) -> (x = y?=w297:bool)
        n115 = Equal?(x=w324, y=w325) -> (x = y?=w298:bool)
        n116 = Number To Boolean Array(number=w308) -> (Boolean array=w307:bool[])
        n117 = Or(x=w297, y=w298) -> (x .or. y?=w296:bool)
        n118 = Split 1D Array(array=w307, index=w305) -> (first subarray=w306:bool[])  [unwired: 1 out]
        n119 = Index Array(array=w306, index #1=1) -> (element #1=w299:bool, element #2=w300:bool)  [unwired: 1 in]
        n120 = Or(x=w299, y=w300) -> ()  [unwired: 1 out]
        n121 = case shown="True" w296 {
          tunnel: w297 -> [_ w340]
          tunnel: w298 -> [_ _]
          tunnel: w316 -> [_ w339]
          tunnel: [w333 w338] -> w310
          tunnel: w319 -> [w332 w337]
          tunnel: [w332 w336] -> w314
          tunnel: w301 -> [w331 w334]
          tunnel: [w331 w335] -> w312
          frame False {
            w333 = bool[] [FALSE, TRUE, FALSE, FALSE, TRUE, FALSE, FALSE, FALSE, FALSE, FALSE, FALSE, FALSE, FALSE, FALSE, FALSE, FALSE, FALSE, FALSE, FALSE, FALSE, FALSE, FALSE, FALSE, FALSE, FALSE, FALSE, FALSE, FALSE, FALSE, FALSE, FALSE, FALSE]  # HOSUING & MECH WRONG CODE
            # "WRONG SCANEED DATA"
          }
          frame True {
            # "SCANNED DATA CORRECT"
            n122 = case shown="True" w340 {
              tunnel: w339 -> [w341 w347]
              tunnel: [w345 w350] -> w338
              tunnel: w337 -> [w344 w349]
              tunnel: [w343 w348] -> w336
              tunnel: w334 -> [w342 w346]
              tunnel: [w342 w346] -> w335
              frame False {
                w345 = bool[] [TRUE, FALSE, FALSE, FALSE, FALSE, FALSE, FALSE, FALSE, FALSE, FALSE, FALSE, FALSE, FALSE, FALSE, FALSE, FALSE, FALSE, FALSE, FALSE, FALSE, FALSE, FALSE, FALSE, FALSE, FALSE, FALSE, FALSE, FALSE, FALSE, FALSE, FALSE, FALSE]  # MECH OK
                # "MECHANISUM"
                n123 = Bundle By Name(cluster=w344, "CYCLE DATA.SCANNED MECHANISUM ST1"=w341) -> (w343:T2)
              }
              frame True {
                w350 = bool[] [FALSE, FALSE, FALSE, TRUE, FALSE, FALSE, FALSE, FALSE, FALSE, FALSE, FALSE, FALSE, FALSE, FALSE, FALSE, FALSE, FALSE, FALSE, FALSE, FALSE, FALSE, FALSE, FALSE, FALSE, FALSE, FALSE, FALSE, FALSE, FALSE, FALSE, FALSE, FALSE]  # HOSU OK
                # "HOUSING"
                n124 = Bundle By Name(cluster=w349, "CYCLE DATA.SCANNED HOUSING ST1"=w347) -> (w348:T2)
              }
            }
          }
        }
        n125 = call "TAT_PLC_Data_WRITE_2_INT.vi"("Enum"=w313, "error in (no error)"=w312, "Array"=w310) -> ("error out"=w311:errorcluster)  [unwired: 7 in, 1 out]
      }
      frame "STATION_1_CMPLT_OK" {
        w351 = ""
        n126 = Unbundle By Name(w357) -> ("CYCLE DATA.SCANNED HOUSING 1 OK"=w356:string[], "CYCLE DATA.SCANNED HOUSING ST1"=w355:string)
        n127 = Build Array (concatenate)(w356, w355) -> (w354:string[])
        n128 = Bundle By Name(cluster=w357, "CYCLE DATA.SCANNED HOUSING 1 OK"=w354) -> (w353:T2)
        n129 = Bundle By Name(cluster=w353, "CYCLE DATA.SCANNED MECHANISUM ST1"=w351, "CYCLE DATA.SCANNED HOUSING ST1"=w351) -> (w352:T2)
        n130 = local write "MECHANISUM DATA ST1"(w351) -> ()
        n131 = local write "HOUSING DATA ST1"(w351) -> ()
        n132 = local write "Scaned 1 Code"(w351) -> ()
      }
      frame "STATION_1_ABORT_NG" {
        w359 = ""
        n133 = Bundle By Name(cluster=w361, "CYCLE DATA.SCANNED MECHANISUM ST1"=w359, "CYCLE DATA.SCANNED HOUSING ST1"=w359) -> (w360:T2)
        n134 = local write "MECHANISUM DATA ST1"(w359) -> ()
        n135 = local write "HOUSING DATA ST1"(w359) -> ()
        n136 = local write "Scaned 1 Code"(w359) -> ()
      }
      frame "AUTO_CYC_START_ST2" {
        w366 = 0
        w369 = dbl[] []
        w371 = ""
        w373 = enum16{"Int", "Update"}."Int"  # Enum
        n137 = Unbundle By Name(w363) -> ("REFERENCE.TRIP FORCE"=w368:refnum<vi>, "REFERENCE.RESET FORCE"=w367:refnum<vi>)
        n138 = property on="Property Node" class="DigNum (strict)"(reference=w367, "Value"=w366, "NumText.BGColor"=u32 16777226) -> ()  [unwired: 1 in, 2 out]
        n139 = property on="Property Node" class="DigNum (strict)"(reference=w368, "Value"=w366, "NumText.BGColor"=u32 16777226) -> ()  [unwired: 1 in, 2 out]
        n140 = Bundle By Name(cluster=w363, "CYCLE DATA.SCANNED HOUSING TF ST2"=w371, "CYCLE DATA.X DISTANCE"=w369, "CYCLE DATA.Y LOAD"=w369) -> (w372:T2)
        n141 = call "debug_csv_graph_values.vi"("error in"=w375, "Enum"=w373) -> ("error our"=w374:errorcluster)  [unwired: 2 in, 1 out]
        n142 = Bundle(w369, w369) -> (w370:cluster{dbl[], dbl[]})  [unwired: 1 in]
        n143 = local write "TF RUNNING PART ST2"(w371) -> ()
        n144 = local write "LOAD gms"(w370) -> ()
      }
      frame "SCAN_STATION_2" {
        w381 = enum16{"Read", "Write"}."Write"  # Enum
        w390 = 16  # index
        w389 = enum16{"Read", "Write"}."Read"  # Enum
        # "COMPARE WITH\nSTATION 1 SCANNED CODE \nWHICH VALIDATE PART DONE ON\nSTATION 1"
        n145 = flat-sequence {
          tunnel: [w415] -> w397
          tunnel: w395 -> [w415]
          tunnel: [w414] -> w396
          tunnel: [w418] -> w387
          tunnel: w397 -> [w418]
          tunnel: [w417] -> w378
          tunnel: w396 -> [w417]
          frame #0 {
            n146 = local read "Scaned 2 Code"() -> (w414:string)
          }
          frame #1 {
            n147 = local write "Scaned 2 Code"("") -> ()
          }
        }
        n148 = Unbundle By Name(w376) -> ("CYCLE DATA.SCANNED HOUSING 1 OK"=w385:string[])
        n149 = call "TAT_PLC_Data_read_INT.vi"("Enum"=w389, "error in (no error)"=w387) -> ("error out"=w386:errorcluster, "Array 2"=w394:u16[])  [unwired: 8 in]
        n150 = Search 1D Array(1D array=w385, element=w378) -> (index of element=w384:i32)  [unwired: 1 in]
        n151 = Index Array(array=w394) -> (element=w393:u16)  [unwired: 1 in]
        n152 = Number To Boolean Array(number=w393) -> (Boolean array=w392:bool[])
        n153 = Not Equal?(x=w384, y=-1) -> (x != y?=w382:bool)
        n154 = Split 1D Array(array=w392, index=w390) -> (first subarray=w391:bool[])  [unwired: 1 out]
        n155 = Index Array(array=w391, index=8) -> ()  [unwired: 1 out]
        n156 = case shown="False" w382 {
          selector: w382 -> [w401 _]
          tunnel: [w400 w412] -> w380
          tunnel: [w402 w413] -> w379
          tunnel: w386 -> [w403 w413]
          tunnel: w378 -> [_ w410]
          tunnel: [w399 w411] -> w377
          tunnel: w376 -> [w399 w409]
          frame False {
            # "STATION 2 SCAN FAIL"
            n157 = case shown="True" w401 {
              tunnel: w403 -> [w405 w408]
              tunnel: [w405 w407] -> w402
              tunnel: [w404 w406] -> w400
              frame False {
                w404 = bool[] [FALSE, FALSE, FALSE, FALSE, FALSE, FALSE, TRUE, FALSE, FALSE, FALSE, FALSE, FALSE, FALSE, FALSE, FALSE, FALSE, FALSE, FALSE, FALSE, FALSE, FALSE, FALSE, FALSE, FALSE, FALSE, FALSE, FALSE, FALSE, FALSE, FALSE, FALSE, FALSE]  # STATION 1 DNT DONE
                # "PREVIOUS STATION DNT DONE"
              }
              frame True {
                w406 = bool[] [FALSE, FALSE, FALSE, FALSE, FALSE, FALSE, TRUE, FALSE, FALSE, FALSE, FALSE, FALSE, FALSE, FALSE, FALSE, FALSE, FALSE, FALSE, FALSE, FALSE, FALSE, FALSE, FALSE, FALSE, FALSE, FALSE, FALSE, FALSE, FALSE, FALSE, FALSE, FALSE]  # STATION 1 DNT DONE
                # "HOUSE CODE NOT MATCHED WITH STATION 1"
                n158 = Merge Errors(w408) -> (w407:errorcluster)
              }
            }
          }
          frame True {
            w412 = bool[] [FALSE, FALSE, FALSE, FALSE, FALSE, FALSE, FALSE, FALSE, FALSE, FALSE, FALSE, FALSE, FALSE, FALSE, TRUE, FALSE, FALSE, FALSE, FALSE, FALSE, FALSE, FALSE, FALSE, FALSE, FALSE, FALSE, FALSE, FALSE, FALSE, FALSE, FALSE, FALSE]  # STATION 1 DONE  AND HOUSE MATCH
            # "OK"
            n159 = Bundle By Name(cluster=w409, "CYCLE DATA.SCANNED HOUSING TF ST2"=w410) -> (w411:T2)
          }
        }
        n160 = call "TAT_PLC_Data_WRITE_2_INT.vi"("Enum"=w381, "error in (no error)"=w379, "Array"=w380) -> ("error out"=w398:errorcluster)  [unwired: 7 in, 1 out]
      }
      frame "LOAD CELL PICK UP" {
        n161 = local read "Load Cell Scaned"() -> (w420:string)
        n162 = call "IN_RANGE_CHECKING.vi"("error in (no error)"=w424, "Load Cell Scaned"=w420, "AUTO CYC DATA in"=w421) -> ("error out"=w425:errorcluster, "Cluster"=→"LOAD gms":cluster{dbl[], dbl[]}, "AUTO CYC DATA out"=w422:T2, "Enum"=→"TRIP CAUSE":T1)  [unwired: 5 in]
      }
      frame "PRINT" {
        w434 = 4  # index
        w430 = enum16{"Read", "Write"}."Read"  # Enum
        # "TRIP FORCE LOWER LIMIT FAIL\t%1$S\nTRIP FORCE HIGER LIMIT FAIL\t%2$S\nTRIP RESET FORCE LOWER LIMIT FAIL\t%3$S\nTRIP RESET FORCE HIGER LIMIT FAIL\t%4$S"
        n163 = call "TAT_PLC_Data_read_INT.vi"("Enum"=w430, "error in (no error)"=w429) -> ("error out"=w428:errorcluster, "Array 2"=w431:u16[])  [unwired: 8 in]
        n164 = Index Array(array=w431, index=1) -> (element=w432:u16)
        n165 = Number To Boolean Array(number=w432) -> (Boolean array=w433:bool[])
        n166 = Split 1D Array(array=w433, index=w434) -> (first subarray=w426:bool[])  [unwired: 1 out]
        n167 = for {
          tunnel: string[] ["TRIP FORCE LOWER LIMIT FAIL NG", "TRIP FORCE HIGER LIMIT FAIL", "TRIP RESET FORCE LOWER LIMIT FAIL", "TRIP RESET FORCE HIGER LIMIT FAIL"] -> [w459] mode=indexing
          tunnel: [w458] -> w440 mode=indexing
          tunnel: w426 -> [w460] mode=indexing
          n168 = Select(t=w459, s=w460, f="") -> (s? t:f=w458:string)
        }
        n169 = Unbundle By Name(w442) -> ("CYCLE DATA.prn DATA"=w441:string)
        n170 = TCP Open Connection(address=w444, remote port or service name=u16 9100, timeout ms (60000)=5000, error in (no error)=w428) -> (connection ID=w449:refnum<k5>, error out=w455:errorcluster)  [unwired: 1 in]
        n171 = Index Array(array=w440) -> (element #1=w439:string, element #2=w438:string, element #3=w437:string, element #4=w436:string)  [unwired: 4 in]
        n172 = call "Stall Data Flow.vim"("value in"=w455, "milliseconds to wait"=u32 200) -> ("value out"=w450:errorcluster)  [unwired: 1 out]
        n173 = Format Into String(format string=w441, w439, w438, w437, w436) -> (resulting string=w435:string)  [unwired: 2 in, 1 out]
        n174 = TCP Write(connection ID=w449, data in=w435, error in (no error)=w450, 9:5000 ("timeout ms (60000)")) -> (connection ID out=w447:refnum<k5>, error out=w448:errorcluster)  [unwired: 1 out]
        n175 = call "Stall Data Flow.vim"("value in"=w448, "milliseconds to wait"=u32 200) -> ("value out"=w456:errorcluster)  [unwired: 1 out]
        n176 = TCP Close Connection(connection ID=w447, error in (no error)=w456) -> (error out=w445:errorcluster)  [unwired: 2 out]
      }
      frame "AUTO_CYCLE_COMP_ST2" {
        w461 = dbl[] []
        w462 = ""
        # "COMPARE WITH\nSTATION 1 SCANNED CODE \nWHICH VALIDATE PART DONE ON\nSTATION 1"
        n177 = Unbundle By Name(w463) -> ("CYCLE DATA.SCANNED HOUSING 1 OK"=w467:string[], "CYCLE DATA.SCANNED HOUSING TF ST2"=w469:string)
        n178 = Search 1D Array(1D array=w467, element=w469) -> (index of element=w466:i32)  [unwired: 1 in]
        n179 = Not Equal?(x=w466, y=-1) -> (x != y?=w468:bool)
        n180 = case shown="True" w468 {
          tunnel: w467 -> [_ w477]
          tunnel: w466 -> [_ w476]
          tunnel: [w472 w473] -> w465
          tunnel: w463 -> [w472 w475]
          frame False {
          }
          frame True {
            n181 = Delete From Array(array=w477, index=w476) -> (array with subset deleted=w474:string[])  [unwired: 1 in, 1 out]
            n182 = Bundle By Name(cluster=w475, "CYCLE DATA.SCANNED HOUSING 1 OK"=w474) -> (w473:T2)
          }
        }
        n183 = Bundle By Name(cluster=w465, "CYCLE DATA.SCANNED HOUSING TF ST2"=w462, "CYCLE DATA.X DISTANCE"=w461, "CYCLE DATA.Y LOAD"=w461) -> (w464:T2)
        n184 = local write "TF RUNNING PART ST2"(w462) -> ()
        n185 = local write "Scaned 2 Code"(w462) -> ()
      }
      frame "AUTO_CYCLE_ABORT_ST2" {
        w478 = dbl[] []
        w479 = ""
        n186 = Bundle By Name(cluster=w480, "CYCLE DATA.SCANNED HOUSING TF ST2"=w479, "CYCLE DATA.X DISTANCE"=w478, "CYCLE DATA.Y LOAD"=w478) -> (w481:T2)
        n187 = local write "TF RUNNING PART ST2"(w479) -> ()
        n188 = local write "Scaned 2 Code"(w479) -> ()
      }
      frame "Error_Handler" {
        w484 = T3 2 items=["no dialog", "OK message", "continue or stop message", "OK message + warnings", "continue/stop + warnings"]  # type of dialog (OK msg:1)
        n189 = call <vilib>:"Simple Error Handler.vi"("type of dialog (OK msg:1)"=w484, "error in (no error)"=w486) -> ("error out"=w485:errorcluster)  [unwired: 3 in, 4 out]
      }
      frame "Stop" {
        w490 = enum16{"Read", "Write"}."Write"  # Enum
        w492 = enum16{"Read", "Write"}."Write"  # Enum
        w496 = QUEUE_STATES."CLOSE Q"  # QUEUE ST
        # "STOP"
        n190 = call "TAT_PLC_Data_WRITE_1_INT.vi"("Enum"=w492, "error in (no error)"=w497, "Array"=bool[] [FALSE, FALSE, FALSE, FALSE, FALSE, FALSE, FALSE]) -> ("error out"=w488:errorcluster)  [unwired: 7 in, 1 out]
        n191 = call "TAT_PLC_Data_WRITE_2_INT.vi"("Enum"=w490, "error in (no error)"=w497, "Array"=bool[] [FALSE, FALSE, FALSE, FALSE, FALSE, FALSE, FALSE, FALSE, FALSE, FALSE, FALSE, FALSE, FALSE, FALSE, FALSE, FALSE, FALSE, FALSE, FALSE, FALSE, FALSE, FALSE, FALSE, FALSE, FALSE, FALSE, FALSE, FALSE, FALSE, FALSE, FALSE, FALSE]) -> ("error out"=w487:errorcluster)  [unwired: 7 in, 1 out]
        n192 = call "AUTO_Queue_States.vi"("QUEUE ST"=w496, "error in"=w497) -> ("error OUT"=w493:errorcluster)  [unwired: 8 in, 1 out]
        n193 = Merge Errors(w488, w487, w493) -> (w494:errorcluster)
      }
    }
    "MAIN LOOP STOPED ?" <- w69
    n194 = Get Date/Time String(want seconds? (F)=FALSE) -> (date string=w73:string, time string=w72:string)  [unwired: 2 in]
    n195 = case shown="Error" w64 {
      selector: w64 -> [w76 w79]
      tunnel: [w76 w78] -> w63
      frame No Error {
      }
      frame Error {
        w77 = T6[] [enum."Error_Handler"] items=["Int", "Int2", "CLUSTER_UPDATE", "WAIT", "AUTO_CYCLE_RUNNING_ST1", "SCAN_STATION_1", "STATION_1_CMPLT_OK", "STATION_1_ABORT_NG", "SCAN_STATION_2", "LOAD CELL PICK UP", "AUTO_CYCLE_COMP_ST2", "AUTO_CYCLE_ABORT_ST2", "PRINT", "CYCLE_DISTANCE FAIL_ST2", "AUTO_CYC_START_ST2", "Error_Handler", "Stop"]  # AUTO ST IN
        w80 = QUEUE_STATES."EN Q"  # QUEUE ST
        n196 = call "AUTO_Queue_States.vi"("QUEUE ST"=w80, "error in"=w79, "AUTO ST IN"=w77) -> ("error OUT"=w78:errorcluster)  [unwired: 7 in, 1 out]
      }
    }
    n197 = Concatenate Strings(w73, "\n", w72) -> (→"DATE/TIME":string)
    n198 = Wait (ms)(milliseconds to wait=u32 150) -> ()  [unwired: 1 out]
  }
  n199 = Unbundle By Name(w2) -> ("LOAD CELL COM"=w24:refnum<visa-resource-name>)
  n200 = Unbundle By Name(w2) -> ("SCAN 2 COM"=w10:refnum<visa-resource-name>)
  n201 = Unbundle By Name(w2) -> ("SCAN 1 COM"=w25:refnum<visa-resource-name>)
  n202 = call <vilib>:"Clear Errors.vi"("error in (no error)"=w22) -> ("error out"=w33:errorcluster)  [unwired: 5 in, 1 out]
  n203 = while {
    tunnel: w33 -> [w502]
    tunnel: [w515] -> _
    tunnel: w31 -> [w514]
    shift-right: [w513] -> _
    shift-left: "" -> [w522]
    shift-right: [w521] -> _
    shift-left: string[] [] ("Alarms") -> [w523]
    tunnel: [w501] -> w32
    stop <- w503 stop-if-true
    w508 = 16
    w499 = enum16{"Read", "Write"}."Read"  # Enum
    # "ALARM"
    n204 = call "TAT_PLC_Data_read_INT.vi"("Enum"=w499, "error in (no error)"=w502) -> ("error out"=w501:errorcluster, "Array 2"=w500:u16[])  [unwired: 8 in]
    n205 = Index Array(array=w500, index #1=9) -> (element #1=w511:u16, element #2=w510:u16)  [unwired: 1 in]
    n206 = Number To Boolean Array(number=w511) -> (Boolean array=w509:bool[])
    n207 = Number To Boolean Array(number=w510) -> (Boolean array=w507:bool[])
    n208 = Split 1D Array(array=w509, index=w508) -> (first subarray=w506:bool[])  [unwired: 1 out]
    n209 = Split 1D Array(array=w507, index=w508) -> (first subarray=w505:bool[])  [unwired: 1 out]
    n210 = Build Array (concatenate)(w506, w505) -> (w504:bool[])
    n211 = flat-sequence {
      tunnel: [w528] -> w517
      tunnel: [w530] -> w521
      tunnel: w514 -> [w529]
      tunnel: w501 -> [w528]
      tunnel: w504 -> [w527]
      frame #0 {
        n212 = for {
          tunnel: w527 -> [w535] mode=indexing
          tunnel: [w531] -> w530 mode=indexing
          tunnel: w529 -> [w533]
          i -> [w534]
          n213 = case shown="False" w535 {
            tunnel: w534 -> [_ w541]
            tunnel: [-1 w541] -> w532
            frame False {
            }
            frame True {
            }
          }
          n214 = case shown="0, Default" w532 {
            selector: w532 -> [w537 _]
            tunnel: w533 -> [w538 _]
            tunnel: [w536 ""] -> w531
            frame 0, Default {
              n215 = Index Array(array=w538, index=w537) -> (element=w536:string)
            }
            frame -1 {
            }
          }
        }
      }
    }
    n216 = call <vilib>:"Clear Errors.vi"("error in (no error)"=w517) -> ("error out"=w516:errorcluster)  [unwired: 5 in, 1 out]
    n217 = Not Equal?(x=w521, y=w523) -> (x != y?=w525:bool[])
    n218 = First Call?() -> (First Call?: T/F=w520:bool)
    n219 = Or Array Elements(Boolean array=w525) -> (logical OR=w519:bool)
    n220 = Or(x=w519, y=w520) -> (x .or. y?=w518:bool)
    n221 = case shown="True" w518 {
      tunnel: [w543 w545] -> w524
      tunnel: w522 -> [w543 _]
      tunnel: w521 -> [_ w546]
      tunnel: w516 -> [w542 w544]
      tunnel: [w542 w544] -> w515
      frame False {
      }
      frame True {
        # "Load new meassage list"
        n222 = for {
          tunnel: w546 -> [w549] mode=indexing
          shift-right: [w551] -> w545
          shift-left: "" -> [w550]
          n223 = Empty String/Path?(string/path=w549) -> (empty?=w548:bool)
          n224 = case shown="True" w548 {
            tunnel: [w554 w557] -> w551
            tunnel: w550 -> [w553 w556]
            tunnel: w549 -> [w552 _]
            frame False {
              n225 = Concatenate Strings(w553, w552) -> (w554:string)
            }
            frame True {
              n226 = call <vilib>:"Space Constant.vi"() -> ("String"=w555:string)
              n227 = Concatenate Strings(w556, w555) -> (w557:string)
            }
          }
        }
      }
    }
    n228 = local read "MAIN LOOP STOPED ?"() -> (w503:bool)
    n229 = Rotate String(1:w524) -> (0:w513:string)
    "ALARMS:-" <- w513
    n230 = Wait (ms)(milliseconds to wait=u32 100) -> ()  [unwired: 1 out]
    "Alarms" <- w521
  }
  n231 = while {
    shift-right: [w565] -> w9
    shift-left: _ -> [w567]
    shift-right: [w563] -> _
    shift-left: enum16{"Ini", "scanning", "Close"}."Ini" -> [w564]
    shift-right: [w562] -> w6
    shift-left: _ -> [w561]
    tunnel: w10 -> [w558]
    stop <- w560 stop-if-true
    # "Scanner Loop 2"
    n232 = case shown="No Error" w567 {
      selector: w567 -> [w574 w607]
      tunnel: [w573 w606] -> w565
      tunnel: w564 -> [w572 _]
      tunnel: [w571 enum16{"Ini", "scanning", "Close"}."scanning"] -> w563
      tunnel: [w570 w604] -> w562
      tunnel: w561 -> [w569 w604]
      tunnel: w558 -> [w568 _]
      frame No Error {
        n233 = case shown="\"scanning\", Default" w572 {
          tunnel: w574 -> [w581 w589]
          tunnel: [w579 w592] -> w573
          tunnel: [enum16{"Ini", "scanning", "Close"}."scanning" enum16{"Ini", "scanning", "Close"}."scanning"] -> w571
          tunnel: [w578 w591] -> w570
          tunnel: w569 -> [_ w587]
          tunnel: w568 -> [w580 _]
          frame "Ini" {
            w576 = u8 10  # Termination Character
            w577 = u32 1000  # timeout
            n234 = call-poly "VISA Configure Serial Port"("VISA resource name"=w580, "timeout (10sec)"=w577, "termination char\n(0xA = '\\n' = LF)"=w576, "Enable Termination\nChar (T)"=TRUE, "error in (no error)"=w581) -> ("VISA resource name out"=w578:refnum<visa-resource-name>, "error out"=w579:errorcluster)  [unwired: 9 in]
          }
          frame "scanning", Default {
            w583 = 1073676294  # ON PORT LENTHG READ
            n235 = property class="Instr"(reference=w587, error in=w589) -> (reference out=w586:refnum<visa-resource-name>, error out=w588:errorcluster, "Bytes at Port"=w584:u32)
            n236 = Not Equal To 0?(x=w584) -> (x != 0?=w585:bool)
            n237 = case shown="True" w585 {
              tunnel: [w595 w601] -> w591
              tunnel: [w594 w600] -> w590
              tunnel: w588 -> [w594 w599]
              tunnel: w586 -> [w595 w598]
              tunnel: w584 -> [_ w597]
              frame False {
              }
              frame True {
                n238 = VISA Read(VISA resource name=w598, byte count=w597, error in (no error)=w599) -> (VISA resource name out=w601:refnum<visa-resource-name>, read buffer=w596:string, error out=w600:errorcluster)  [unwired: 1 out]
                n239 = local write "Scaned 2 Code"(w596) -> ()
              }
            }
            n240 = call <vilib>:"Clear Errors.vi"("error in (no error)"=w590, "specific error code to clear (0: all)"=w583) -> ("error out"=w592:errorcluster)  [unwired: 4 in, 1 out]
          }
        }
      }
      frame Error {
        w602 = T3 2 items=["no dialog", "OK message", "continue or stop message", "OK message + warnings", "continue/stop + warnings"] ("type of dialog (OK msg:1)")
        n241 = call <vilib>:"Simple Error Handler.vi"("type of dialog (OK msg:1)"=w602, "error in (no error)"=w607) -> ("error out"=w603:errorcluster)  [unwired: 3 in, 4 out]
        n242 = call <vilib>:"Clear Errors.vi"("error in (no error)"=w603) -> ("error out"=w606:errorcluster)  [unwired: 5 in, 1 out]
      }
    }
    n243 = local read "MAIN LOOP STOPED ?"() -> (w566:bool)
    n244 = Or(x=w565, y=w566) -> (x .or. y?=w560:bool)
    "Scanner 2 Status" <- w560
    n245 = Wait (ms)(milliseconds to wait=u32 500) -> ()  [unwired: 1 out]
  }
  n246 = while {
    shift-right: [w615] -> w29
    shift-left: w22 -> [w617]
    shift-right: [w613] -> _
    shift-left: enum16{"Ini", "scanning", "Close"}."Ini" -> [w614]
    shift-right: [w612] -> w17
    shift-left: _ -> [w611]
    tunnel: w25 -> [w608]
    stop <- w610 stop-if-true
    # "Scanner Loop 1"
    n247 = case shown="No Error" w617 {
      selector: w617 -> [w624 w657]
      tunnel: [w623 w656] -> w615
      tunnel: w614 -> [w622 _]
      tunnel: [w621 enum16{"Ini", "scanning", "Close"}."scanning"] -> w613
      tunnel: [w620 w654] -> w612
      tunnel: w611 -> [w619 w654]
      tunnel: w608 -> [w618 _]
      frame No Error {
        n248 = case shown="\"scanning\", Default" w622 {
          tunnel: w624 -> [w631 w639]
          tunnel: [w629 w642] -> w623
          tunnel: [enum16{"Ini", "scanning", "Close"}."scanning" enum16{"Ini", "scanning", "Close"}."scanning"] -> w621
          tunnel: [w628 w641] -> w620
          tunnel: w619 -> [_ w637]
          tunnel: w618 -> [w630 _]
          frame "Ini" {
            w626 = u8 10  # Termination Character
            w627 = u32 1000  # timeout
            n249 = call-poly "VISA Configure Serial Port"("VISA resource name"=w630, "timeout (10sec)"=w627, "termination char\n(0xA = '\\n' = LF)"=w626, "Enable Termination\nChar (T)"=TRUE, "error in (no error)"=w631) -> ("VISA resource name out"=w628:refnum<visa-resource-name>, "error out"=w629:errorcluster)  [unwired: 9 in]
          }
          frame "scanning", Default {
            w633 = 1073676294  # ON PORT LENTHG READ
            n250 = property class="Instr"(reference=w637, error in=w639) -> (reference out=w636:refnum<visa-resource-name>, error out=w638:errorcluster, "Bytes at Port"=w634:u32)
            n251 = Not Equal To 0?(x=w634) -> (x != 0?=w635:bool)
            n252 = case shown="True" w635 {
              tunnel: [w645 w651] -> w641
              tunnel: [w644 w650] -> w640
              tunnel: w638 -> [w644 w649]
              tunnel: w636 -> [w645 w648]
              tunnel: w634 -> [_ w647]
              frame False {
              }
              frame True {
                n253 = VISA Read(VISA resource name=w648, byte count=w647, error in (no error)=w649) -> (VISA resource name out=w651:refnum<visa-resource-name>, read buffer=w646:string, error out=w650:errorcluster)  [unwired: 1 out]
                n254 = global write "PLC_to_Auto.vi" "scanner data"(w646) -> ()
                n255 = local write "Scaned 1 Code"(w646) -> ()
              }
            }
            n256 = call <vilib>:"Clear Errors.vi"("error in (no error)"=w640, "specific error code to clear (0: all)"=w633) -> ("error out"=w642:errorcluster)  [unwired: 4 in, 1 out]
          }
        }
      }
      frame Error {
        w652 = T3 2 items=["no dialog", "OK message", "continue or stop message", "OK message + warnings", "continue/stop + warnings"] ("type of dialog (OK msg:1)")
        n257 = call <vilib>:"Simple Error Handler.vi"("type of dialog (OK msg:1)"=w652, "error in (no error)"=w657) -> ("error out"=w653:errorcluster)  [unwired: 3 in, 4 out]
        n258 = call <vilib>:"Clear Errors.vi"("error in (no error)"=w653) -> ("error out"=w656:errorcluster)  [unwired: 5 in, 1 out]
      }
    }
    n259 = local read "MAIN LOOP STOPED ?"() -> (w616:bool)
    n260 = Or(x=w615, y=w616) -> (x .or. y?=w610:bool)
    "Scanner 1 Status" <- w610
    n261 = Wait (ms)(milliseconds to wait=u32 500) -> ()  [unwired: 1 out]
  }
  n262 = while {
    shift-right: [w659] -> w19
    shift-left: w22 -> [w667]
    shift-right: [w664] -> _
    shift-left: enum16{"Ini", "scanning", "Close"}."Ini" -> [w665]
    shift-right: [w663] -> w18
    shift-left: _ -> [w662]
    tunnel: w24 -> [w660]
    stop <- w666 stop-if-true
    # "Load Cell  Loop"
    n263 = case shown="No Error" w667 {
      selector: w667 -> [w674 w723]
      tunnel: [w673 w725] -> w659
      tunnel: w665 -> [w672 _]
      tunnel: [w671 enum16{"Ini", "scanning", "Close"}."Ini"] -> w664
      tunnel: [w670 w721] -> w663
      tunnel: w662 -> [w669 w721]
      tunnel: w660 -> [w668 _]
      frame No Error {
        n264 = case shown="\"Ini\"" w672 {
          tunnel: w674 -> [w682 w688]
          tunnel: [w680 w689] -> w673
          tunnel: [enum16{"Ini", "scanning", "Close"}."scanning" enum16{"Ini", "scanning", "Close"}."scanning"] -> w671
          tunnel: [w679 w685] -> w670
          tunnel: w669 -> [_ w687]
          tunnel: w668 -> [w681 _]
          frame "Ini" {
            w675 = TRUE  # Enable Termination Char (T)
            w676 = u8 10  # termination char (0xA = '\n' = LF)
            w677 = u32 9600  # baud rate (115200)
            w678 = u32 1000  # timeout
            n265 = call-poly "VISA Configure Serial Port"("VISA resource name"=w681, "timeout (10sec)"=w678, "termination char\n(0xA = '\\n' = LF)"=w676, "Enable Termination\nChar (T)"=w675, "baud rate (9600)"=w677, "error in (no error)"=w682) -> ("VISA resource name out"=w679:refnum<visa-resource-name>, "error out"=w680:errorcluster)  [unwired: 8 in]
          }
          frame "scanning", Default {
            n266 = disable-structure shown="Enabled" {
              disable-tunnel: w688 -> [w701 w719]
              disable-tunnel: w687 -> [w699 w718]
              disable-tunnel: [w694 w712] -> w686
              disable-tunnel: [w692 w710] -> w685
              disable-tunnel: [w691 w715] -> w684
              frame Disabled {
                w691 = 1073676294  # ON PORT LENTHG READ
                n267 = property class="Instr"(reference=w699, error in=w701) -> (reference out=w698:refnum<visa-resource-name>, error out=w700:errorcluster, "Bytes at Port"=w696:u32)
                n268 = Not Equal To 0?(x=w696) -> (x != 0?=w697:bool)
                n269 = case shown="True" w697 {
                  tunnel: [w703 w709] -> w693
                  tunnel: [w702 w708] -> w695
                  tunnel: w700 -> [w702 w707]
                  tunnel: w698 -> [w703 w706]
                  tunnel: w696 -> [_ w704]
                  frame False {
                  }
                  frame True {
                    n270 = VISA Read(VISA resource name=w706, byte count=w704, error in (no error)=w707) -> (VISA resource name out=w709:refnum<visa-resource-name>, read buffer=w705:string, error out=w708:errorcluster)  [unwired: 1 out]
                    n271 = local write "Load Cell Scaned"(w705) -> ()
                  }
                }
                n272 = VISA Clear(VISA resource name=w693, error in (no error)=w695) -> (VISA resource name out=w692:refnum<visa-resource-name>, error out=w694:errorcluster)
              }
              frame Enabled {
                w715 = -1073807339  # BYTE SIZE READ
                n273 = VISA Read(VISA resource name=w718, byte count=u32 300, error in (no error)=w719) -> (VISA resource name out=w711:refnum<visa-resource-name>, read buffer=w716:string, error out=w713:errorcluster)  [unwired: 1 out]
                n274 = Empty String/Path?(string/path=w716) -> (empty?=w717:bool)
                n275 = case shown="False" w717 {
                  tunnel: w716 -> [w720 _]
                  frame False {
                    n276 = local write "Load Cell Scaned"(w720) -> ()
                  }
                  frame True {
                  }
                }
                n277 = VISA Clear(VISA resource name=w711, error in (no error)=w713) -> (VISA resource name out=w710:refnum<visa-resource-name>, error out=w712:errorcluster)
              }
            }
            n278 = call <vilib>:"Clear Errors.vi"("error in (no error)"=w686, "specific error code to clear (0: all)"=w684) -> ("error out"=w689:errorcluster)  [unwired: 4 in, 1 out]
          }
        }
      }
      frame Error {
        n279 = VISA Close(VISA resource name=w721, error in (no error)=w723) -> (error out=w722:errorcluster)
        n280 = call <vilib>:"Clear Errors.vi"("error in (no error)"=w722) -> ("error out"=w725:errorcluster)  [unwired: 5 in, 1 out]
      }
    }
    n281 = local read "MAIN LOOP STOPED ?"() -> (w666:bool)
    n282 = Unbundle By Name(w659) -> ("status"=→"Load Cell Status":bool)
    n283 = Wait (ms)(milliseconds to wait=u32 900) -> ()  [unwired: 1 out]
  }
  n284 = call <vilib>:"Clear Errors.vi"("error in (no error)"=w19) -> ("error out"=w20:errorcluster)  [unwired: 5 in, 1 out]
  n285 = call <vilib>:"Clear Errors.vi"("error in (no error)"=w9) -> ("error out"=w7:errorcluster)  [unwired: 5 in, 1 out]
  n286 = call <vilib>:"Clear Errors.vi"("error in (no error)"=w29) -> ("error out"=w16:errorcluster)  [unwired: 5 in, 1 out]
  n287 = VISA Close(VISA resource name=w18, error in (no error)=w20) -> (error out=w5:errorcluster)
  n288 = VISA Close(VISA resource name=w6, error in (no error)=w7) -> (error out=w4:errorcluster)
  n289 = VISA Close(VISA resource name=w17, error in (no error)=w16) -> (error out=w15:errorcluster)
  "error out 2" <- w15
  n290 = Merge Errors(w5, w4, w15, w32, w48) -> (w47:errorcluster)
  n291 = call <vilib>:"Simple Error Handler.vi"("type of dialog (OK msg:1)"=w44, "error in (no error)"=w47) -> ("error out"=w40:errorcluster)  [unwired: 3 in, 4 out]
  "error out" <- w40
  n292 = call <vilib>:"Clear Errors.vi"("error in (no error)"=w40) -> ("error out"=w36:errorcluster)  [unwired: 5 in, 1 out]
  n293 = flat-sequence {
    tunnel: w36 -> [_]
    frame #0 {
      n294 = global write "PLC_to_Auto.vi" "AUTO SCREEN ON"(FALSE) -> ()
    }
  }
  n295 = property class="App"() -> ("App.Kind"=w43:T8)  [unwired: 2 in, 2 out]
  n296 = Merge Errors(w36) -> (w41:errorcluster)
  n297 = case shown="\"Run Time System\"" w43 {
    tunnel: w41 -> [_ w728]
    frame "invalid app kind", Default {
    }
    frame "Run Time System" {
      n298 = call <vilib>:"Clear Errors.vi"("error in (no error)"=w728) -> ("error out"=w727:errorcluster)  [unwired: 5 in, 1 out]
      n299 = invoke class="VI" method="FP.Close"(error in=w727) -> ()  [unwired: 2 in, 3 out]
    }
  }
